vi "rsidr_core_global.vi"() -> ()   [LabVIEW 2015, in "Rohde&Schwarz CMXP Base.lvlib"]
doc: "This Global variable contains driver's:\n- Attributes\n- Range Tables\n- Repeated Capabilities"
uses:
  <instrlib>/Rohde&Schwarz CMXP Base/Rohde&Schwarz CMXP Base.lvlib
  <instrlib>/Rohde&Schwarz CMXP Base/Private/rsidr_core.llb/type_Input_Format_Attribute.ctl
  <instrlib>/Rohde&Schwarz CMXP Base/Private/rsidr_core.llb/type_Input_Format_RangeTable.ctl
  <instrlib>/Rohde&Schwarz CMXP Base/Private/rsidr_core.llb/type_Input_Format_RepCap.ctl
  <instrlib>/Rohde&Schwarz CMXP Base/Private/rsidr_core.llb/rsidr_core.lvlib
panel:
  in  "Repeated Capabilities":T1[](array[typedef])=[{"repCapName"="i", "indetifiers"=["chan1", "chan2", "chan3", "chan4", "chan5", "chan6", "chan7", "chan8", "chan9", "chan10", "chan11", "chan12", "chan13", "chan14", "chan15", "chan16", "chan17", "chan18", "chan19", "chan20", "chan21", "chan22", "chan23", "chan24", "chan25", "chan26", "chan27", "chan28", "chan29", "chan30", "chan31", "chan32"], "cmdValues"=["1", "2", "3", "4", "5", "6", "7", "8", "9", "10", "11", "12", "13", "14", "15", "16", "17", "18", "19", "20", "21", "22", "23", "24", "25", "26", "27", "28", "29", "30", "31", "32"]}]
  in  "Range Tables":T2[](array[typedef])=[{"Type"=2, "Name"="rsCmxpBase_rngMeasurementMode", "Entries"=[{"Name"="IQ", "Value 1"=0.0, "Value 2"=0.0, "Command"="IQ"}, {"Name"="Level", "Value 1"=1.0, "Value 2"=0.0, "Command"="LEV"}, {"Name"="Verify IQ", "Value 1"=2.0, "Value 2"=0.0, "Command"="VIQ"}]}, {"Type"=2, "Name"="rsCmxpBase_rngMode", "Entries"=[{"Name"="All", "Value 1"=0.0, "Value 2"=0.0, "Command"="ALL"}, {"Name"="Wtime", "Value 1"=1.0, "Value 2"=0.0, "Command"="WTI"}]}, {"Type"=2, "Name"="rsCmxpBase_rngOptionType", "Entries"=[{"Name"="All", "Value 1"=0.0, "Value 2"=0.0, "Command"="ALL"}, {"Name"="SW Option", "Value 1"=1.0, "Value 2"=0.0, "Command"="SWOP"}, {"Name"="HW Option", "Value 1"=2.0, "Value 2"=0.0, "Command"="HWOP"}, {"Name"="SW Package", "Value 1"=3.0, "Value 2"=0.0, "Command"="SWP"}, {"Name"="FWA", "Value 1"=4.0, "Value 2"=0.0, "Command"="FWA"}]}, {"Type"=2, "Name"="rsCmxpBase_rngValidity", "Entries"=[{"Name"="All", "Value 1"=0.0, "Value 2"=0.0, "Command"="ALL"}, {"Name"="Valid", "Value 1"=1.0, "Value 2"=0.0, "Command"="VAL"}, {"Name"="Functional", "Value 1"=2.0, "Value 2"=0.0, "Command"="FUNC"}]}, {"Type"=0, "Name"="rsCmxpBase_rngPortNumber", "Entries"=[{"Name"="", "Value 1"=0.0, "Value 2"=32767.0, "Command"=""}]}, {"Type"=0, "Name"="rsCmxpBase_rngTimer", "Entries"=[{"Name"="", "Value 1"=0.0, "Value 2"=inf, "Command"=""}]}, {"Type"=2, "Name"="rsCmxpBase_rngAuthenticationAlgorithm", "Entries"=[{"Name"="Milenage", "Value 1"=0.0, "Value 2"=0.0, "Command"="MIL"}, {"Name"="XOR", "Value 1"=1.0, "Value 2"=0.0, "Command"="XOR"}]}, {"Type"=2, "Name"="rsCmxpBase_rngOperatorCode", "Entries"=[{"Name"="Ciphered", "Value 1"=0.0, "Value 2"=0.0, "Command"="CIPH"}, {"Name"="Plain", "Value 1"=1.0, "Value 2"=0.0, "Command"="PLA"}]}, {"Type"=2, "Name"="rsCmxpBase_rngSelectFrequencyFormat", "Entries"=[{"Name"="Internal", "Value 1"=0.0, "Value 2"=0.0, "Command"="INTernal"}, {"Name"="External", "Value 1"=1.0, "Value 2"=0.0, "Command"="EXTernal"}]}, {"Type"=0, "Name"="rsCmxpBase_rngReferenceFrequencySettings", "Entries"=[{"Name"="", "Value 1"=1000000.0, "Value 2"=80000000.0, "Command"=""}]}, {"Type"=2, "Name"="rsCmxpBase_rngProtocolMode", "Entries"=[{"Name"="Raw", "Value 1"=0.0, "Value 2"=0.0, "Command"="RAW"}, {"Name"="Agilent", "Value 1"=1.0, "Value 2"=0.0, "Command"="AGIL"}, {"Name"="IEEE1147", "Value 1"=2.0, "Value 2"=0.0, "Command"="IEEE1174"}]}, {"Type"=2, "Name"="rsCmxpBase_rngQueryMeasurementState", "Entries"=[{"Name"="Off", "Value 1"=0.0, "Value 2"=0.0, "Command"="OFF"}, {"Name"="Run", "Value 1"=1.0, "Value 2"=0.0, "Command"="RUN"}, {"Name"="Ready", "Value 1"=2.0, "Value 2"=0.0, "Command"="RDY"}]}, {"Type"=2, "Name"="rsCmxpBase_rngQueryLastMeasurmentMode", "Entries"=[{"Name"="Invalid", "Value 1"=0.0, "Value 2"=0.0, "Command"="INV"}, {"Name"="Passed", "Value 1"=1.0, "Value 2"=0.0, "Command"="PASS"}, {"Name"="Progress", "Value 1"=2.0, "Value 2"=0.0, "Command"="PROG"}, {"Name"="Failed", "Value 1"=3.0, "Value 2"=0.0, "Command"="FAIL"}, {"Name"="Skipped", "Value 1"=4.0, "Value 2"=0.0, "Command"="SKIP"}, {"Name"="Not A Value", "Value 1"=5.0, "Value 2"=0.0, "Command"="NAV"}]}, {"Type"=2, "Name"="rsCmxpBase_rngRemoteTraceHeaderFilter", "Entries"=[{"Name"="All", "Value 1"=0.0, "Value 2"=0.0, "Command"="ALL"}, {"Name"="Line ID", "Value 1"=1.0, "Value 2"=0.0, "Command"="LID"}, {"Name"="Event Yype", "Value 1"=2.0, "Value 2"=0.0, "Command"="ETYP"}, {"Name"="Time Stamp", "Value 1"=3.0, "Value 2"=0.0, "Command"="TST"}, {"Name"="Duration", "Value 1"=4.0, "Value 2"=0.0, "Command"="DUR"}, {"Name"="VISA Resource", "Value 1"=5.0, "Value 2"=0.0, "Command"="VRES"}, {"Name"="Instrument Number", "Value 1"=6.0, "Value 2"=0.0, "Command"="TENV"}, {"Name"="Connection", "Value 1"=7.0, "Value 2"=0.0, "Command"="CONN"}, {"Name"="Data", "Value 1"=8.0, "Value 2"=0.0, "Command"="DATA"}]}, {"Type"=2, "Name"="rsCmxpBase_rngRemoteTraceTarget", "Entries"=[{"Name"="Screen", "Value 1"=0.0, "Value 2"=0.0, "Command"="SCR"}, {"Name"="File", "Value 1"=1.0, "Value 2"=0.0, "Command"="FILE"}, {"Name"="Screen and file", "Value 1"=2.0, "Value 2"=0.0, "Command"="SAF"}]}, {"Type"=2, "Name"="rsCmxpBase_rngDUTBandRestrictionTXConnector", "Entries"=[{"Name"="None", "Value 1"=0.0, "Value 2"=0.0, "Command"="NONE"}, {"Name"="One", "Value 1"=1.0, "Value 2"=0.0, "Command"="ONE"}]}, {"Type"=2, "Name"="rsCmxpBase_rngDUTBandRestrictionRXConnector", "Entries"=[{"Name"="None", "Value 1"=0.0, "Value 2"=0.0, "Command"="NONE"}, {"Name"="One", "Value 1"=1.0, "Value 2"=0.0, "Command"="ONE"}, {"Name"="Two", "Value 1"=2.0, "Value 2"=0.0, "Command"="TWO"}]}, {"Type"=2, "Name"="rsCmxpBase_rngDUTControlMode", "Entries"=[{"Name"="Manual", "Value 1"=0.0, "Value 2"=0.0, "Command"="MAN"}, {"Name"="Automatic", "Value 1"=1.0, "Value 2"=0.0, "Command"="AUTO"}]}, {"Type"=2, "Name"="rsCmxpBase_rngUSIMLengthXOR", "Entries"=[{"Name"="Any", "Value 1"=0.0, "Value 2"=0.0, "Command"="ANY"}, {"Name"="L04", "Value 1"=1.0, "Value 2"=0.0, "Command"="L04"}, {"Name"="L05", "Value 1"=2.0, "Value 2"=0.0, "Command"="L05"}, {"Name"="L06", "Value 1"=3.0, "Value 2"=0.0, "Command"="L06"}, {"Name"="L07", "Value 1"=4.0, "Value 2"=0.0, "Command"="L07"}, {"Name"="L08", "Value 1"=5.0, "Value 2"=0.0, "Command"="L08"}, {"Name"="L09", "Value 1"=6.0, "Value 2"=0.0, "Command"="L09"}, {"Name"="L10", "Value 1"=7.0, "Value 2"=0.0, "Command"="L10"}, {"Name"="L11", "Value 1"=8.0, "Value 2"=0.0, "Command"="L11"}, {"Name"="L12", "Value 1"=9.0, "Value 2"=0.0, "Command"="L12"}, {"Name"="L13", "Value 1"=10.0, "Value 2"=0.0, "Command"="L13"}, {"Name"="L14", "Value 1"=11.0, "Value 2"=0.0, "Command"="L14"}, {"Name"="L15", "Value 1"=12.0, "Value 2"=0.0, "Command"="L15"}, {"Name"="L16", "Value 1"=13.0, "Value 2"=0.0, "Command"="L16"}]}, {"Type"=2, "Name"="rsCmxpBase_rngDUTPowerCycleState", "Entries"=[{"Name"="Ready", "Value 1"=0.0, "Value 2"=0.0, "Command"="RDY"}, {"Name"="Run", "Value 1"=1.0, "Value 2"=0.0, "Command"="RUN"}]}, {"Type"=2, "Name"="rsCmxpBase_rngDataFormat", "Entries"=[{"Name"="ASCII", "Value 1"=0.0, "Value 2"=0.0, "Command"="ASC"}, {"Name"="Real", "Value 1"=1.0, "Value 2"=0.0, "Command"="REAL"}, {"Name"="Binary", "Value 1"=2.0, "Value 2"=0.0, "Command"="BIN"}, {"Name"="Hexadecimal", "Value 1"=3.0, "Value 2"=0.0, "Command"="HEX"}, {"Name"="Octal", "Value 1"=4.0, "Value 2"=0.0, "Command"="OCT"}]}, {"Type"=2, "Name"="rsCmxpBase_rngSeverity", "Entries"=[{"Name"="Info", "Value 1"=0.0, "Value 2"=0.0, "Command"="INFO"}, {"Name"="Warning", "Value 1"=1.0, "Value 2"=0.0, "Command"="WARN"}, {"Name"="Error", "Value 1"=2.0, "Value 2"=0.0, "Command"="ERR"}]}, {"Type"=2, "Name"="rsCmxpBase_rngTriggerDirection", "Entries"=[{"Name"="In", "Value 1"=0.0, "Value 2"=0.0, "Command"="IN"}, {"Name"="Out", "Value 1"=1.0, "Value 2"=0.0, "Command"="OUT"}]}, {"Type"=2, "Name"="rsCmxpBase_rngTriggerSlope", "Entries"=[{"Name"="Rising Edge", "Value 1"=0.0, "Value 2"=0.0, "Command"="REDG"}, {"Name"="Falling Edge", "Value 1"=1.0, "Value 2"=0.0, "Command"="FEDG"}]}, {"Type"=2, "Name"="rsCmxpBase_rngTriggerConnectorCatalogNameStyle", "Entries"=[{"Name"="Default", "Value 1"=0.0, "Value 2"=0.0, "Command"="NAME"}, {"Name"="Fully Qualified Name", "Value 1"=1.0, "Value 2"=0.0, "Command"="FQN"}, {"Name"="Label Only", "Value 1"=2.0, "Value 2"=0.0, "Command"="LNAM"}]}, {"Type"=2, "Name"="rsCmxpBase_rngDUTBandRestrictionType", "Entries"=[{"Name"="LTE", "Value 1"=0.0, "Value 2"=0.0, "Command"="LTE"}, {"Name"="New Radio", "Value 1"=1.0, "Value 2"=0.0, "Command"="NRAD"}]}, {"Type"=2, "Name"="rsCmxpBase_rngDUTBandTX", "Entries"=[{"Name"="TX0", "Value 1"=0.0, "Value 2"=0.0, "Command"="TX0"}, {"Name"="TX1", "Value 1"=1.0, "Value 2"=0.0, "Command"="TX1"}, {"Name"="None", "Value 1"=2.0, "Value 2"=0.0, "Command"="NONE"}]}, {"Type"=2, "Name"="rsCmxpBase_rngDUTBandRX", "Entries"=[{"Name"="RX0", "Value 1"=0.0, "Value 2"=0.0, "Command"="RX0"}, {"Name"="RX1", "Value 1"=1.0, "Value 2"=0.0, "Command"="RX1"}, {"Name"="RX2", "Value 1"=2.0, "Value 2"=0.0, "Command"="RX2"}, {"Name"="RX3", "Value 1"=3.0, "Value 2"=0.0, "Command"="RX3"}, {"Name"="None", "Value 1"=4.0, "Value 2"=0.0, "Command"="NONE"}]}, {"Type"=2, "Name"="rsCmxpBase_rngDUTBandType", "Entries"=[{"Name"="LTE", "Value 1"=0.0, "Value 2"=0.0, "Command"="LTE"}, {"Name"="New Radio", "Value 1"=1.0, "Value 2"=0.0, "Command"="NRAD"}, {"Name"="WLAN", "Value 1"=2.0, "Value 2"=0.0, "Command"="WLAN"}]}, {"Type"=2, "Name"="rsCmxpBase_rngDUTControlAutomationFramework", "Entries"=[{"Name"="External Automation Application", "Value 1"=0.0, "Value 2"=0.0, "Command"="EXT"}]}, {"Type"=2, "Name"="rsCmxpBase_rngRemoteTraceLogRows", "Entries"=[{"Name"="Latest", "Value 1"=0.0, "Value 2"=0.0, "Command"="LAT"}, {"Name"="List", "Value 1"=1.0, "Value 2"=0.0, "Command"="LIST"}, {"Name"="Error", "Value 1"=2.0, "Value 2"=0.0, "Command"="ERR"}, {"Name"="Connection", "Value 1"=3.0, "Value 2"=0.0, "Command"="CONN"}]}, {"Type"=2, "Name"="rsCmxpBase_rngRemoteTraceEvents", "Entries"=[{"Name"="All", "Value 1"=0.0, "Value 2"=0.0, "Command"="ALL"}, {"Name"="Input", "Value 1"=1.0, "Value 2"=0.0, "Command"="INP"}, {"Name"="Output", "Value 1"=2.0, "Value 2"=0.0, "Command"="OUTP"}, {"Name"="Error", "Value 1"=3.0, "Value 2"=0.0, "Command"="ERR"}, {"Name"="Connection", "Value 1"=4.0, "Value 2"=0.0, "Command"="CONN"}, {"Name"="Duration", "Value 1"=5.0, "Value 2"=0.0, "Command"="DUR"}, {"Name"="Remote Local", "Value 1"=6.0, "Value 2"=0.0, "Command"="RLOC"}]}, {"Type"=2, "Name"="rsCmxpBase_rngRFConnectionDirection", "Entries"=[{"Name"="RX", "Value 1"=0.0, "Value 2"=0.0, "Command"="RX"}, {"Name"="TX", "Value 1"=1.0, "Value 2"=0.0, "Command"="TX"}, {"Name"="TX & RX", "Value 1"=2.0, "Value 2"=0.0, "Command"="RXTX"}]}, {"Type"=0, "Name"="rsCmxpBase_rngSystemDataFormat", "Entries"=[{"Name"="", "Value 1"=0.0, "Value 2"=0.0, "Command"=""}]}, {"Type"=2, "Name"="rsCmxpBase_rngActiveDUTActionState", "Entries"=[{"Name"="Ready", "Value 1"=0.0, "Value 2"=0.0, "Command"="RDY"}, {"Name"="Run", "Value 1"=1.0, "Value 2"=0.0, "Command"="RUN"}]}, {"Type"=2, "Name"="rsCmxpBase_rngActiveDUTMobileAction", "Entries"=[{"Name"="Reject", "Value 1"=0.0, "Value 2"=0.0, "Command"="REJ"}, {"Name"="Disconnect", "Value 1"=1.0, "Value 2"=0.0, "Command"="DISC"}, {"Name"="Accept", "Value 1"=2.0, "Value 2"=0.0, "Command"="ACC"}, {"Name"="Connect", "Value 1"=3.0, "Value 2"=0.0, "Command"="CONN"}]}] {"Type" items=["Range", "Coerced", "Discrete"]}
  in  "Attributes":T3[](array[typedef])=[{"Level"=1, "Class Only"=TRUE, "Identifier"="", "Descriptive Name"="Base", "Data Type"=0, "Command"="", "Access"=0, "Range Table"="", "Read Callback"="", "Write Callback"="", "Supported Models"="", "Instrument Options"="", "Flags"=0, "Help"="Contains functionality to configure the base R&S Radio Communication Tester."}, {"Level"=2, "Class Only"=TRUE, "Identifier"="", "Descriptive Name"="Macro", "Data Type"=0, "Command"="", "Access"=0, "Range Table"="", "Read Callback"="", "Write Callback"="", "Supported Models"="", "Instrument Options"="", "Flags"=0, "Help"="The following remote control commands are related to macro files and macro execution."}, {"Level"=3, "Class Only"=FALSE, "Identifier"="RSCMXPBASE_ATTR_CREATE_MACRO", "Descriptive Name"="Create Macro", "Data Type"=6, "Command"="*DMC", "Access"=2, "Range Table"="", "Read Callback"="", "Write Callback"="", "Supported Models"="", "Instrument Options"="", "Flags"=0, "Help"="Creates a macro. If the label exists already, the macro contents are overwritten. Macros are deleted when a remote connection is closed but can be saved to a macro file for later reuse, see MMEMory:STORe:MACRo. Avoid using labels which are identical with supported remote control commands.  In contrast to SCPI stipulations, remote commands have priority over macros.\n\nAvailable Repeated Capabilities:\nNone\n\nRemote-control command(s):\n*DMC"}, {"Level"=3, "Class Only"=FALSE, "Identifier"="RSCMXPBASE_ATTR_MACRO_EXECUTION_STATE", "Descriptive Name"="Macro Execution State", "Data Type"=3, "Command"="*EMC", "Access"=2, "Range Table"="", "Read Callback"="", "Write Callback"="", "Supported Models"="", "Instrument Options"="", "Flags"=0, "Help"="Enables or disables the execution of all macros that are defined for the active remote connection. Note: In contrast to SCPI specifications, macro execution is disabled by default.\n\nAvailable Repeated Capabilities:\nNone\n\nRemote-control command(s):\n*EMC"}, {"Level"=3, "Class Only"=FALSE, "Identifier"="RSCMXPBASE_ATTR_HIDDEN_QUERY_MACRO", "Descriptive Name"="Query Macro", "Data Type"=2, "Command"="*GMC?", "Access"=0, "Range Table"="", "Read Callback"="", "Write Callback"="", "Supported Models"="", "Instrument Options"="", "Flags"=8, "Help"="Returns the contents of a macro.\n\nAvailable Repeated Capabilities:\nNone\n\nRemote-control command(s):\n*GMC?"}, {"Level"=3, "Class Only"=FALSE, "Identifier"="RSCMXPBASE_ATTR_QUERY_MACRO_LABELS", "Descriptive Name"="Query Macro Labels", "Data Type"=2, "Command"="*LMC?", "Access"=0, "Range Table"="", "Read Callback"="", "Write Callback"="", "Supported Models"="", "Instrument Options"="", "Flags"=0, "Help"="Returns the labels of all macros of the active connection.\n\nAvailable Repeated Capabilities:\nNone\n\nRemote-control command(s):\n*LMC?"}, {"Level"=3, "Class Only"=FALSE, "Identifier"="RSCMXPBASE_ATTR_DELETE_ALL_MACROS", "Descriptive Name"="Delete All Macros", "Data Type"=4, "Command"="*PMC", "Access"=1, "Range Table"="", "Read Callback"="", "Write Callback"="", "Supported Models"="", "Instrument Options"="", "Flags"=0, "Help"="Deletes all macros of the active remote connection.\n\nAvailable Repeated Capabilities:\nNone\n\nRemote-control command(s):\n*PMC"}, {"Level"=3, "Class Only"=FALSE, "Identifier"="RSCMXPBASE_ATTR_DELETE_MACRO", "Descriptive Name"="Delete Macro", "Data Type"=2, "Command"="*RMC", "Access"=1, "Range Table"="", "Read Callback"="", "Write Callback"="", "Supported Models"="", "Instrument Options"="", "Flags"=0, "Help"="Deletes a macro.\n\nAvailable Repeated Capabilities:\nNone\n\nRemote-control command(s):\n*RMC"}, {"Level"=3, "Class Only"=FALSE, "Identifier"="RSCMXPBASE_ATTR_LOAD_MACRO", "Descriptive Name"="Load Macro", "Data Type"=6, "Command"="MMEM:LOAD:MACR", "Access"=2, "Range Table"="", "Read Callback"="", "Write Callback"="", "Supported Models"="", "Instrument Options"="", "Flags"=0, "Help"="Creates a macro, reading the macro contents from a file. If the label exists already, the macro contents are overwritten.\nAvoid using labels which are identical with supported remote control commands.  In contrast to SCPI stipulations, remote commands have priority over macros.\n\nAvailable Repeated Capabilities:\nNone\n\nRemote-control command(s):\nMMEMory:LOAD:MACRo"}, {"Level"=3, "Class Only"=FALSE, "Identifier"="RSCMXPBASE_ATTR_SAVE_MACRO", "Descriptive Name"="Save Macro", "Data Type"=6, "Command"="MMEM:STOR:MACR", "Access"=1, "Range Table"="", "Read Callback"="", "Write Callback"="", "Supported Models"="", "Instrument Options"="", "Flags"=0, "Help"="Stores the contents of a macro to a file. If the file exists, it is overwritten. If the file does not exist, it is created.\n\nAvailable Repeated Capabilities:\nNone\n\nRemote-control command(s):\nMMEMory:STORe:MACRo"}, {"Level"=3, "Class Only"=FALSE, "Identifier"="RSCMXPBASE_ATTR_START_MACRO_RECORDING", "Descriptive Name"="Start Macro Recording", "Data Type"=2, "Command"="SYST:REC:MACR:FILE:STAR", "Access"=1, "Range Table"="", "Read Callback"="", "Write Callback"="", "Supported Models"="", "Instrument Options"="", "Flags"=0, "Help"="Starts recording of submitted commands into a macro file. If the file exists, it is overwritten. If the file does not exist, it is created.\n\nAvailable Repeated Capabilities:\nNone\n\nRemote-control command(s):\nSYSTem:RECord:MACRo:FILE:STARt"}, {"Level"=3, "Class Only"=FALSE, "Identifier"="RSCMXPBASE_ATTR_STOP_MACRO_RECORDING", "Descriptive Name"="Stop Macro Recording", "Data Type"=4, "Command"="SYST:REC:MACR:FILE:STOP", "Access"=1, "Range Table"="", "Read Callback"="", "Write Callback"="", "Supported Models"="", "Instrument Options"="", "Flags"=0, "Help"="Stops recording of commands into a macro file.\n\nAvailable Repeated Capabilities:\nNone\n\nRemote-control command(s):\nSYSTem:RECord:MACRo:FILE:STOP"}, {"Level"=2, "Class Only"=TRUE, "Identifier"="", "Descriptive Name"="Buffer", "Data Type"=0, "Command"="", "Access"=0, "Range Table"="", "Read Callback"="", "Write Callback"="", "Supported Models"="", "Instrument Options"="", "Flags"=0, "Help"="The following remote control commands are related to response buffers."}, {"Level"=3, "Class Only"=FALSE, "Identifier"="RSCMXPBASE_ATTR_START_BUFFER", "Descriptive Name"="Start Buffer", "Data Type"=2, "Command"="STAR:BASE:BUFF", "Access"=1, "Range Table"="", "Read Callback"="", "Write Callback"="", "Supported Models"="", "Instrument Options"="", "Flags"=0, "Help"="Creates and activates a buffer. If the buffer exists already, it is cleared (equivalent to CLEar:BASE:BUFFer).\n\nAvailable Repeated Capabilities:\nNone\n\nRemote-control command(s):\nSTARt:BASE:BUFFer"}, {"Level"=3, "Class Only"=FALSE, "Identifier"="RSCMXPBASE_ATTR_STOP_BUFFER", "Descriptive Name"="Stop Buffer", "Data Type"=4, "Command"="STOP:BASE:BUFF", "Access"=1, "Range Table"="", "Read Callback"="", "Write Callback"="", "Supported Models"="", "Instrument Options"="", "Flags"=0, "Help"="Deactivates the active buffer. Only one buffer can be active at a time. The buffer and its contents are maintained, but data recording is paused. Use CONTinue:BASE:BUFFer to reactivate a buffer.\n\nAvailable Repeated Capabilities:\nNone\n\nRemote-control command(s):\nSTOP:BASE:BUFFer"}, {"Level"=3, "Class Only"=FALSE, "Identifier"="RSCMXPBASE_ATTR_CONTINUE_BUFFER", "Descriptive Name"="Continue Buffer", "Data Type"=2, "Command"="CONT:BASE:BUFF", "Access"=1, "Range Table"="", "Read Callback"="", "Write Callback"="", "Supported Models"="", "Instrument Options"="", "Flags"=0, "Help"="Reactivates a buffer which was deactivated via STOP:BASE:BUFFer). The R&S CMX500 continues writing data to the buffer.\n\nAvailable Repeated Capabilities:\nNone\n\nRemote-control command(s):\nCONTinue:BASE:BUFFer"}, {"Level"=3, "Class Only"=FALSE, "Identifier"="RSCMXPBASE_ATTR_HIDDEN_FETCH_BUFFER", "Descriptive Name"="Fetch Buffer", "Data Type"=6, "Command"="FETC:BASE:BUFF?", "Access"=0, "Range Table"="", "Read Callback"="", "Write Callback"="", "Supported Models"="", "Instrument Options"="", "Flags"=8, "Help"="Reads the contents of a buffer line. Buffer contents are stored line by line. Every query generates a new buffer line. The queries are not stored together with the results. Reading buffer contents is non-destructive. The lines can be read in arbitrary order.\n\nAvailable Repeated Capabilities:\nNone\n\nRemote-control command(s):\nFETCh:BASE:BUFFer?"}, {"Level"=3, "Class Only"=FALSE, "Identifier"="RSCMXPBASE_ATTR_HIDDEN_FETCH_BUFFER_LINES", "Descriptive Name"="Fetch Buffer Lines", "Data Type"=0, "Command"="FETC:BASE:BUFF:LIN?", "Access"=0, "Range Table"="", "Read Callback"="", "Write Callback"="", "Supported Models"="", "Instrument Options"="", "Flags"=8, "Help"="Returns the number of lines in a buffer.\n\nAvailable Repeated Capabilities:\nNone\n\nRemote-control command(s):\nFETCh:BASE:BUFFer:LINecount?"}, {"Level"=3, "Class Only"=FALSE, "Identifier"="RSCMXPBASE_ATTR_CLEAR_BUFFER", "Descriptive Name"="Clear Buffer", "Data Type"=2, "Command"="CLE:BASE:BUFF", "Access"=1, "Range Table"="", "Read Callback"="", "Write Callback"="", "Supported Models"="", "Instrument Options"="", "Flags"=0, "Help"="Clears the contents of a buffer. You get an empty buffer that you can fill with new commands.\n\nAvailable Repeated Capabilities:\nNone\n\nRemote-control command(s):\nCLEar:BASE:BUFFer"}, {"Level"=3, "Class Only"=FALSE, "Identifier"="RSCMXPBASE_ATTR_DELETE_BUFFER", "Descriptive Name"="Delete Buffer", "Data Type"=2, "Command"="DEL:BASE:BUFF", "Access"=1, "Range Table"="", "Read Callback"="", "Write Callback"="", "Supported Models"="", "Instrument Options"="", "Flags"=0, "Help"="Deletes a buffer.\n\nAvailable Repeated Capabilities:\nNone\n\nRemote-control command(s):\nDELete:BASE:BUFFer"}, {"Level"=2, "Class Only"=TRUE, "Identifier"="", "Descriptive Name"="Timer", "Data Type"=0, "Command"="", "Access"=0, "Range Table"="", "Read Callback"="", "Write Callback"="", "Supported Models"="", "Instrument Options"="", "Flags"=0, "Help"="After execution of a command, it can be necessary to wait a well-defined time before proceeding with command script processing. For example, because the DUT needs some time to stabilize after a modification. Waiting can be achieved using the following commands."}, {"Level"=3, "Class Only"=FALSE, "Identifier"="RSCMXPBASE_ATTR_SET_ABSOLUTE_TIMER", "Descriptive Name"="Set Absolute Timer", "Data Type"=0, "Command"="SYST:TIME:HRT:ABS", "Access"=1, "Range Table"="rsCmxpBase_rngTimer", "Read Callback"="", "Write Callback"="", "Supported Models"="", "Instrument Options"="", "Flags"=1, "Help"="Starts a timer. The timeout is specified relative to an already set timestamp, see RSCMXPBASE_ATTR_SET_TIMESTAMP. When the timer expires, 'Operation Complete' is indicated. This event can be evaluated by polling, via a *OPC? or via *WAI.\n\nAvailable Repeated Capabilities:\nNone\n\nRemote-control command(s):\nSYSTem:TIME:HRTimer:ABSolute"}, {"Level"=3, "Class Only"=FALSE, "Identifier"="RSCMXPBASE_ATTR_SET_RELATIVE_TIMER", "Descriptive Name"="Set Relative Timer", "Data Type"=0, "Command"="SYST:TIME:HRT:REL", "Access"=1, "Range Table"="rsCmxpBase_rngTimer", "Read Callback"="", "Write Callback"="", "Supported Models"="", "Instrument Options"="", "Flags"=1, "Help"="Starts a timer. After the specified timeout, an OPC is generated. When the timer expires, 'Operation Complete' is indicated. This event can be evaluated by polling, via a *OPC? or via *WAI.\n\nAvailable Repeated Capabilities:\nNone\n\nRemote-control command(s):\nSYSTem:TIME:HRTimer:RELative"}, {"Level"=3, "Class Only"=FALSE, "Identifier"="RSCMXPBASE_ATTR_SET_TIMESTAMP", "Descriptive Name"="Set Timestamp", "Data Type"=4, "Command"="SYST:TIME:HRT:ABS:SET", "Access"=1, "Range Table"="", "Read Callback"="", "Write Callback"="", "Supported Models"="", "Instrument Options"="", "Flags"=0, "Help"="This command sets a timestamp with the current system time. A timer can be started with a timeout relative to this timestamp, see SYSTem:TIME:HRTimer:ABSolute. An existing timestamp is overwritten.\n\nAvailable Repeated Capabilities:\nNone\n\nRemote-control command(s):\nSYSTem:TIME:HRTimer:ABSolute:SET"}, {"Level"=3, "Class Only"=FALSE, "Identifier"="RSCMXPBASE_ATTR_QUERY_TIMESTAMP", "Descriptive Name"="Query Timestamp", "Data Type"=2, "Command"="SYST:TIME:HRT:ABS:SET?", "Access"=0, "Range Table"="", "Read Callback"="", "Write Callback"="", "Supported Models"="", "Instrument Options"="", "Flags"=0, "Help"="This command queries a timestamp with the current system time. A query returns seven values, separated by commas:\nYear, month, day, hour, minutes, seconds, milliseconds\n\nAvailable Repeated Capabilities:\nNone\n\nRemote-control command(s):\nSYSTem:TIME:HRTimer:ABSolute:SET?"}, {"Level"=2, "Class Only"=TRUE, "Identifier"="", "Descriptive Name"="DUT", "Data Type"=0, "Command"="", "Access"=0, "Range Table"="", "Read Callback"="", "Write Callback"="", "Supported Models"="", "Instrument Options"="", "Flags"=0, "Help"="Contains settings related to DUTs. Additional DUT settings directly related to signaling are described in the signaling manual.\n\nPrepare DUTs in the library and use exactly one active DUT in the test environment."}, {"Level"=3, "Class Only"=TRUE, "Identifier"="", "Descriptive Name"="Library", "Data Type"=0, "Command"="", "Access"=0, "Range Table"="", "Read Callback"="", "Write Callback"="", "Supported Models"="", "Instrument Options"="", "Flags"=0, "Help"="Contains settings for managing DUTs in a library.\n\nA DUT object has a name, SIM slots, a referenced SIM profile per SIM slot and antenna connectors supporting certain frequency bands."}, {"Level"=4, "Class Only"=FALSE, "Identifier"="RSCMXPBASE_ATTR_DUT_CATALOG", "Descriptive Name"="DUT Catalog", "Data Type"=2, "Command"="CAT:DUT?", "Access"=0, "Range Table"="", "Read Callback"="", "Write Callback"="", "Supported Models"="", "Instrument Options"="", "Flags"=0, "Help"="Queries a list of all DUTs, including inactive DUTs in the library and the active DUT.\n\nAvailable Repeated Capabilities:\nNone\n\nRemote-control command(s):\nCATalog:DUT?"}, {"Level"=4, "Class Only"=FALSE, "Identifier"="RSCMXPBASE_ATTR_DUT_ADD", "Descriptive Name"="DUT Add", "Data Type"=2, "Command"="CRE:DUT", "Access"=1, "Range Table"="", "Read Callback"="", "Write Callback"="", "Supported Models"="", "Instrument Options"="", "Flags"=0, "Help"="Creates a DUT with the specified name.\n\nAssign a unique name to each named object within the test environment. Assigning an already used name can be rejected with an error message, even if the other object has not the same type as the new object.\n\nAvailable Repeated Capabilities:\nNone\n\nRemote-control command(s):\nCREate:DUT"}, {"Level"=4, "Class Only"=FALSE, "Identifier"="RSCMXPBASE_ATTR_HIDDEN_DUT_DUPLICATE", "Descriptive Name"="Hidden DUT Duplicate", "Data Type"=6, "Command"="COPY:DUT", "Access"=1, "Range Table"="", "Read Callback"="", "Write Callback"="", "Supported Models"="", "Instrument Options"="", "Flags"=8, "Help"="Creates a DUT with a new name as a copy of the DUT specified.\n\nAvailable Repeated Capabilities:\nNone\n\nRemote-control command(s):\nCOPY:DUT"}, {"Level"=4, "Class Only"=FALSE, "Identifier"="RSCMXPBASE_ATTR_DUT_DELETE", "Descriptive Name"="DUT Delete", "Data Type"=2, "Command"="DEL:DUT", "Access"=1, "Range Table"="", "Read Callback"="", "Write Callback"="", "Supported Models"="", "Instrument Options"="", "Flags"=0, "Help"="Deletes the DUT with the specified name.\n\nAvailable Repeated Capabilities:\nNone\n\nRemote-control command(s):\nDELete:DUT"}, {"Level"=4, "Class Only"=TRUE, "Identifier"="", "Descriptive Name"="Bands And Connectors", "Data Type"=0, "Command"="", "Access"=0, "Range Table"="", "Read Callback"="", "Write Callback"="", "Supported Models"="", "Instrument Options"="", "Flags"=0, "Help"="Configures the antenna connectors of the inactive DUTs."}, {"Level"=5, "Class Only"=FALSE, "Identifier"="RSCMXPBASE_ATTR_HIDDEN_DUT_CONNECTOR_ADD", "Descriptive Name"="Hidden DUT Connector Add", "Data Type"=6, "Command"="CRE:DUT:PROF:CONN", "Access"=1, "Range Table"="", "Read Callback"="", "Write Callback"="", "Supported Models"="", "Instrument Options"="", "Flags"=8, "Help"="Creates an antenna connector for the inactive DUT.\n\nAssign a unique name to each named object within the test environment. Assigning an already used name can be rejected with an error message, even if the other object has not the same type as the new object.\n\nAvailable Repeated Capabilities:\nNone\n\nRemote-control command(s):\nCREate:DUT:PROFile:CONNector"}, {"Level"=5, "Class Only"=FALSE, "Identifier"="RSCMXPBASE_ATTR_HIDDEN_DUT_CONNECTOR_DELETE", "Descriptive Name"="Hidden DUT Connector Delete", "Data Type"=6, "Command"="DEL:DUT:PROF:CONN", "Access"=1, "Range Table"="", "Read Callback"="", "Write Callback"="", "Supported Models"="", "Instrument Options"="", "Flags"=8, "Help"="Deletes an antenna connector of the inactive DUT.\n\nAvailable Repeated Capabilities:\nNone\n\nRemote-control command(s):\nDELete:DUT:PROFile:CONNector"}, {"Level"=5, "Class Only"=FALSE, "Identifier"="RSCMXPBASE_ATTR_HIDDEN_DUT_CONNECTOR_CATALOG", "Descriptive Name"="Hidden DUT Connector Catalog", "Data Type"=6, "Command"="CAT:DUT:PROF:CONN?", "Access"=0, "Range Table"="", "Read Callback"="", "Write Callback"="", "Supported Models"="", "Instrument Options"="", "Flags"=8, "Help"="Queries a list of all antenna connectors of the inactive DUT.\n\nAvailable Repeated Capabilities:\nNone\n\nRemote-control command(s):\nCATalog:DUT:PROFile:CONNector?"}, {"Level"=5, "Class Only"=FALSE, "Identifier"="RSCMXPBASE_ATTR_HIDDEN_DUT_CONNECTOR_BAND_ADD", "Descriptive Name"="Hidden DUT Connector Band Add", "Data Type"=6, "Command"="ADD:DUT:PROF:CONN:BAND", "Access"=1, "Range Table"="", "Read Callback"="", "Write Callback"="", "Supported Models"="", "Instrument Options"="", "Flags"=8, "Help"="Assigns frequency bands to a single antenna connector of the inactive DUT (connector-centric approach).\n\nYou can assign several bands with a single command. Specify the technology and the band number for each band.\n\nAvailable Repeated Capabilities:\nNone\n\nRemote-control command(s):\nADD:DUT:PROFile:CONNector:BAND"}, {"Level"=5, "Class Only"=FALSE, "Identifier"="RSCMXPBASE_ATTR_HIDDEN_DUT_CONNECTOR_BAND_DELETE", "Descriptive Name"="Hidden DUT Connector Band Delete", "Data Type"=6, "Command"="REM:DUT:PROF:CONN:BAND", "Access"=1, "Range Table"="", "Read Callback"="", "Write Callback"="", "Supported Models"="", "Instrument Options"="", "Flags"=8, "Help"="Removes frequency bands from an antenna connector of the inactive DUT (connector-centric approach).\n\nYou can remove several bands. Specify the technology and the band number for each band.\n\nAvailable Repeated Capabilities:\nNone\n\nRemote-control command(s):\nREMove:DUT:PROFile:CONNector:BAND"}, {"Level"=5, "Class Only"=FALSE, "Identifier"="RSCMXPBASE_ATTR_HIDDEN_DUT_CONNECTOR_BAND_CATALOG", "Descriptive Name"="Hidden DUT Connector Band Catalog", "Data Type"=6, "Command"="CAT:DUT:PROF:CONN:BAND?", "Access"=0, "Range Table"="", "Read Callback"="", "Write Callback"="", "Supported Models"="", "Instrument Options"="", "Flags"=8, "Help"="Queries a list of all frequency bands assigned to an antenna connector of the inactive DUT. Structured according to the connector-centric approach.\n\nThe results are returned as groups of values, with <NoOfBands> pairs of <RatType>, <BandNumber> per group:\n\n{<TX>, <RX>, <NoOfBands>, {<RatType>, <BandNumber>,}<NoOfBands> times} ...\n\nAvailable Repeated Capabilities:\nNone\n\nRemote-control command(s):\nCATalog:DUT:PROFile:CONNector:BAND?"}, {"Level"=4, "Class Only"=TRUE, "Identifier"="", "Descriptive Name"="SIM Slot", "Data Type"=0, "Command"="", "Access"=0, "Range Table"="", "Read Callback"="", "Write Callback"="", "Supported Models"="", "Instrument Options"="", "Flags"=0, "Help"="Manage the SIM slots of inactive DUT objects."}, {"Level"=5, "Class Only"=FALSE, "Identifier"="RSCMXPBASE_ATTR_HIDDEN_DUT_SIM_SLOT_ADD", "Descriptive Name"="Hidden DUT SIM Slot Add", "Data Type"=6, "Command"="CRE:DUT:PROF:SIMS", "Access"=1, "Range Table"="", "Read Callback"="", "Write Callback"="", "Supported Models"="", "Instrument Options"="", "Flags"=8, "Help"="Adds a SIM slot with the assigned SIM profile name to the inactive DUT with the specified name.\n\nAssign a unique name to each named object within the test environment. Assigning an already used name can be rejected with an error message, even if the other object has not the same type as the new object.\n\nAvailable Repeated Capabilities:\nNone\n\nRemote-control command(s):\nCREate:DUT:PROFile:SIMSlot"}, {"Level"=5, "Class Only"=FALSE, "Identifier"="RSCMXPBASE_ATTR_HIDDEN_DUT_SIM_SLOT_DELETE", "Descriptive Name"="Hidden DUT SIM Slot Delete", "Data Type"=6, "Command"="DEL:DUT:PROF:SIMS", "Access"=1, "Range Table"="", "Read Callback"="", "Write Callback"="", "Supported Models"="", "Instrument Options"="", "Flags"=8, "Help"="Deletes the SIM slot with the specified SIM number from the inactive DUT.\n\nAvailable Repeated Capabilities:\nNone\n\nRemote-control command(s):\nDELete:DUT:PROFile:SIMSlot"}, {"Level"=5, "Class Only"=FALSE, "Identifier"="RSCMXPBASE_ATTR_HIDDEN_DUT_SIM_SLOT_CATALOG", "Descriptive Name"="Hidden DUT SIM Slot Catalog", "Data Type"=6, "Command"="CAT:DUT:PROF:SIMS?", "Access"=0, "Range Table"="", "Read Callback"="", "Write Callback"="", "Supported Models"="", "Instrument Options"="", "Flags"=8, "Help"="Queries all SIM slots of the inactive DUT. For each SIM slot, the number and the slot name are returned:\n\n{<SimSlotNo>, <SimProfileName>}1, {...}2, ...\n\nAvailable Repeated Capabilities:\nNone\n\nRemote-control command(s):\nCATalog:DUT:PROFile:SIMSlot?"}, {"Level"=5, "Class Only"=FALSE, "Identifier"="RSCMXPBASE_ATTR_SELECT_DUT_SIM_SLOT", "Descriptive Name"="Select DUT SIM Slot", "Data Type"=0, "Command"="", "Access"=2, "Range Table"="", "Read Callback"="", "Write Callback"="", "Supported Models"="", "Instrument Options"="", "Flags"=0, "Help"="Selects a SIM slot number.\n\nAvailable Repeated Capabilities:\nNone\n\nRemote-control command(s):\n"}, {"Level"=5, "Class Only"=FALSE, "Identifier"="RSCMXPBASE_ATTR_HIDDEN_DUT_SIM_SLOT_PROFILE", "Descriptive Name"="Hidden DUT SIM Slot Profile", "Data Type"=6, "Command"="DUT:PROF:SIMS<SIMSlot>:SIMP", "Access"=2, "Range Table"="", "Read Callback"="rscmxpbase_FormatSIMSlotRepCapRawString_ReadCallback.vi", "Write Callback"="rscmxpbase_FormatSIMSlotRepCapRawString_WriteCallback.vi", "Supported Models"="", "Instrument Options"="", "Flags"=8, "Help"="Assigns the SIM profile to the SlM slot number of the inactive DUT.\n\nAvailable Repeated Capabilities:\nNone\n\nRemote-control command(s):\n[CONFigure:]DUT:PROFile:SIMSlot<no>:SIMProfile"}, {"Level"=5, "Class Only"=FALSE, "Identifier"="RSCMXPBASE_ATTR_HIDDEN_DUT_SIM_SLOT_IMS_SUPPORTED", "Descriptive Name"="Hidden DUT SIM Slot IMS Supported", "Data Type"=6, "Command"="DUT:PROF:SIMS<SIMSlot>:CAP:IMS", "Access"=2, "Range Table"="", "Read Callback"="rscmxpbase_FormatSIMSlotRepCapRawString_ReadCallback.vi", "Write Callback"="rscmxpbase_FormatSIMSlotRepCapRawString_WriteCallback.vi", "Supported Models"="", "Instrument Options"="", "Flags"=8, "Help"="Selects whether the inactive DUT supports IP multimedia subsystem (IMS) services.\n\nAvailable Repeated Capabilities:\nNone\n\nRemote-control command(s):\n[CONFigure:]DUT:PROFile:SIMSlot<no>:CAPability:IMS"}, {"Level"=4, "Class Only"=TRUE, "Identifier"="", "Descriptive Name"="RF Connections", "Data Type"=0, "Command"="", "Access"=0, "Range Table"="", "Read Callback"="", "Write Callback"="", "Supported Models"="", "Instrument Options"="", "Flags"=0, "Help"="For routing, the system handles RF connections, also called \"signal paths\" in remote control."}, {"Level"=5, "Class Only"=FALSE, "Identifier"="RSCMXPBASE_ATTR_HIDDEN_RF_CONNECTION_ADD", "Descriptive Name"="Hidden RF Connection Add", "Data Type"=6, "Command"="CRE:TENV:SPAT", "Access"=1, "Range Table"="", "Read Callback"="", "Write Callback"="", "Supported Models"="", "Instrument Options"="", "Flags"=8, "Help"="Creates a signal path for a selected connector and assigns a name to the path.\n\nAssign a unique name to each named object within the test environment. Assigning an already used name can be rejected with an error message, even if the other object has not the same type as the new object.\n\nAvailable Repeated Capabilities:\nNone\n\nRemote-control command(s):\nCREate:TENVironment:SPATh"}, {"Level"=5, "Class Only"=FALSE, "Identifier"="RSCMXPBASE_ATTR_RF_CONNECTION_DELETE", "Descriptive Name"="RF Connection Delete", "Data Type"=2, "Command"="DEL:TENV:SPAT", "Access"=1, "Range Table"="", "Read Callback"="", "Write Callback"="", "Supported Models"="", "Instrument Options"="", "Flags"=0, "Help"="Deletes a signal path.\n\nAvailable Repeated Capabilities:\nNone\n\nRemote-control command(s):\nDELete:TENVironment:SPATh"}, {"Level"=5, "Class Only"=FALSE, "Identifier"="RSCMXPBASE_ATTR_RF_CONNECTION_CATALOG", "Descriptive Name"="RF Connection Catalog", "Data Type"=2, "Command"="CAT:TENV:SPAT?", "Access"=0, "Range Table"="", "Read Callback"="", "Write Callback"="", "Supported Models"="", "Instrument Options"="", "Flags"=0, "Help"="Returns all signal path names.\n\nAvailable Repeated Capabilities:\nNone\n\nRemote-control command(s):\nCATalog:TENVironment:SPATh?"}, {"Level"=5, "Class Only"=FALSE, "Identifier"="RSCMXPBASE_ATTR_HIDDEN_RF_CONNECTION_INFORMATION", "Descriptive Name"="Hidden RF Connection Information", "Data Type"=6, "Command"="TENV:SPAT:INFO?", "Access"=0, "Range Table"="", "Read Callback"="", "Write Callback"="", "Supported Models"="", "Instrument Options"="", "Flags"=8, "Help"="Returns information about the specified signal path.\n\nAvailable Repeated Capabilities:\nNone\n\nRemote-control command(s):\n[CONFigure:]TENVironment:SPATh:INFO?"}, {"Level"=5, "Class Only"=FALSE, "Identifier"="RSCMXPBASE_ATTR_HIDDEN_SIGNAL_PATH_DIRECTION", "Descriptive Name"="Hidden Signal Path Direction", "Data Type"=6, "Command"="TENV:SPAT:DIR", "Access"=2, "Range Table"="", "Read Callback"="", "Write Callback"="", "Supported Models"="", "Instrument Options"="", "Flags"=8, "Help"="Defines the direction of a signal path (TX/RX of the instrument).\n\nAvailable Repeated Capabilities:\nNone\n\nRemote-control command(s):\n[CONFigure:]TENVironment:SPATh:DIRection"}, {"Level"=3, "Class Only"=TRUE, "Identifier"="", "Descriptive Name"="Active DUT", "Data Type"=0, "Command"="", "Access"=0, "Range Table"="", "Read Callback"="", "Write Callback"="", "Supported Models"="", "Instrument Options"="", "Flags"=0, "Help"="Configures seetings of active DUT used in the test environment."}, {"Level"=4, "Class Only"=FALSE, "Identifier"="RSCMXPBASE_ATTR_DUT_ACTIVE", "Descriptive Name"="DUT Active", "Data Type"=2, "Command"="SENS:DUT:ACT?", "Access"=0, "Range Table"="", "Read Callback"="", "Write Callback"="", "Supported Models"="", "Instrument Options"="", "Flags"=0, "Help"="Queries the name of the active DUT.\n\nAvailable Repeated Capabilities:\nNone\n\nRemote-control command(s):\nSENSe:DUT:ACTive?"}, {"Level"=4, "Class Only"=FALSE, "Identifier"="RSCMXPBASE_ATTR_DUT_ACTIVATE", "Descriptive Name"="DUT Activate", "Data Type"=2, "Command"="ACT:DUT", "Access"=1, "Range Table"="", "Read Callback"="", "Write Callback"="", "Supported Models"="", "Instrument Options"="", "Flags"=0, "Help"="Activates the DUT with the specified name for usage in the test environment.\n\nAvailable Repeated Capabilities:\nNone\n\nRemote-control command(s):\nACTivate:DUT"}, {"Level"=4, "Class Only"=FALSE, "Identifier"="RSCMXPBASE_ATTR_SELECT_ACTIVE_DUT_SIM_SLOT", "Descriptive Name"="Select Active DUT SIM Slot", "Data Type"=0, "Command"="", "Access"=2, "Range Table"="", "Read Callback"="", "Write Callback"="", "Supported Models"="", "Instrument Options"="", "Flags"=0, "Help"="Selects a SIM slot number for the active DUT.\n\nAvailable Repeated Capabilities:\nNone\n\nRemote-control command(s):\n"}, {"Level"=4, "Class Only"=TRUE, "Identifier"="", "Descriptive Name"="Band Restrictions", "Data Type"=0, "Command"="", "Access"=0, "Range Table"="", "Read Callback"="", "Write Callback"="", "Supported Models"="", "Instrument Options"="", "Flags"=0, "Help"="Downscales the number of used TX and RX DUT connectors for a specific test session."}, {"Level"=5, "Class Only"=FALSE, "Identifier"="RSCMXPBASE_ATTR_ACTIVE_DUT_BAND_RESTRICTIONS_ENABLED", "Descriptive Name"="Active DUT Band Restrictions Enabled", "Data Type"=3, "Command"="DUT:BAND:REST:ENAB", "Access"=2, "Range Table"="", "Read Callback"="", "Write Callback"="", "Supported Models"="", "Instrument Options"="", "Flags"=0, "Help"="Enables restrictions on the number of used DUT connectors for the active DUT.\n\nAvailable Repeated Capabilities:\nNone\n\nRemote-control command(s):\n[CONFigure:]DUT:BAND:RESTrictions:ENABle"}, {"Level"=5, "Class Only"=FALSE, "Identifier"="RSCMXPBASE_ATTR_ACTIVE_DUT_BAND_RESTRICTIONS_CATALOG", "Descriptive Name"="Active DUT Band Restrictions Catalog", "Data Type"=2, "Command"="CAT:DUT:BAND:REST?", "Access"=0, "Range Table"="", "Read Callback"="", "Write Callback"="", "Supported Models"="", "Instrument Options"="", "Flags"=0, "Help"="Queries the DUT connector restrictions for the active DUT.\n\nAvailable Repeated Capabilities:\nNone\n\nRemote-control command(s):\nCATalog:DUT:BAND:RESTrictions?"}, {"Level"=5, "Class Only"=FALSE, "Identifier"="RSCMXPBASE_ATTR_HIDDEN_ACTIVE_DUT_BAND_RESTRICTIONS", "Descriptive Name"="Hidden Active DUT Band Restrictions", "Data Type"=6, "Command"="DUT:BAND:REST", "Access"=2, "Range Table"="", "Read Callback"="", "Write Callback"="", "Supported Models"="", "Instrument Options"="", "Flags"=8, "Help"="Configures restrictions for a frequency band assigned to connectors of the active DUT.\n\nAvailable Repeated Capabilities:\nNone\n\nRemote-control command(s):\n[CONFigure:]DUT:BAND:RESTrictions"}, {"Level"=4, "Class Only"=TRUE, "Identifier"="", "Descriptive Name"="Runtime Parameters", "Data Type"=0, "Command"="", "Access"=0, "Range Table"="", "Read Callback"="", "Write Callback"="", "Supported Models"="", "Instrument Options"="", "Flags"=0, "Help"="Contains functionality to query runtime parameters reported by the active DUT."}, {"Level"=5, "Class Only"=FALSE, "Identifier"="RSCMXPBASE_ATTR_ACTIVE_DUT_IMS_SUPPORT_ENABLED", "Descriptive Name"="Active DUT IMS Support Enabled", "Data Type"=3, "Command"="DUT:SIMS<ActiveDUTSIMSlot>:UEC:IMS", "Access"=2, "Range Table"="", "Read Callback"="rscmxpbase_FormatActiveSIMSlotRepCapBoolean_ReadCallback.vi", "Write Callback"="rscmxpbase_FormatActiveSIMSlotRepCapBoolean_WriteCallback.vi", "Supported Models"="", "Instrument Options"="", "Flags"=0, "Help"="Selects whether the active DUT supports IP multimedia subsystem (IMS) services.\n\nAvailable Repeated Capabilities:\nNone\n\nRemote-control command(s):\n[CONFigure:]DUT:SIMSlot<SimSlotIdx>:UECapability:IMS"}, {"Level"=5, "Class Only"=FALSE, "Identifier"="RSCMXPBASE_ATTR_ACTIVE_DUT_IMS", "Descriptive Name"="Active DUT IMS", "Data Type"=3, "Command"="SENS:DUT:MOD<ActiveDUTSIMSlot>:CAP:REP:IMS?", "Access"=0, "Range Table"="", "Read Callback"="rscmxpbase_FormatActiveSIMSlotRepCapBoolean_ReadCallback.vi", "Write Callback"="rscmxpbase_FormatActiveSIMSlotRepCapBoolean_WriteCallback.vi", "Supported Models"="", "Instrument Options"="", "Flags"=0, "Help"="Queries the reported IMS capabilities of the active DUT.\n\nAvailable Repeated Capabilities:\nNone\n\nRemote-control command(s):\nSENSe:DUT:MODem<ModemIdx>:CAPability:REPorted:IMS?"}, {"Level"=5, "Class Only"=FALSE, "Identifier"="RSCMXPBASE_ATTR_ACTIVE_DUT_IMEI", "Descriptive Name"="Active DUT IMEI", "Data Type"=2, "Command"="SENS:DUT:MOD<ActiveDUTSIMSlot>:CAP:REP:IMEI?", "Access"=0, "Range Table"="", "Read Callback"="rscmxpbase_FormatActiveSIMSlotRepCapString_ReadCallback.vi", "Write Callback"="rscmxpbase_FormatActiveSIMSlotRepCapString_WriteCallback.vi", "Supported Models"="", "Instrument Options"="", "Flags"=0, "Help"="Queries the reported IMEI of the active DUT.\n\nAvailable Repeated Capabilities:\nNone\n\nRemote-control command(s):\nSENSe:DUT:MODem<ModemIdx>:CAPability:REPorted:IMEI?"}, {"Level"=4, "Class Only"=TRUE, "Identifier"="", "Descriptive Name"="SIM Slot", "Data Type"=0, "Command"="", "Access"=0, "Range Table"="", "Read Callback"="", "Write Callback"="", "Supported Models"="", "Instrument Options"="", "Flags"=0, "Help"="Manages the SIM slots of the active DUT. Each SIM slot has an assigned SIM profile."}, {"Level"=5, "Class Only"=FALSE, "Identifier"="RSCMXPBASE_ATTR_ACTIVE_DUT_SIM_SLOT_ADD", "Descriptive Name"="Active DUT SIM Slot Add", "Data Type"=2, "Command"="CRE:DUT:SIMS", "Access"=1, "Range Table"="", "Read Callback"="", "Write Callback"="", "Supported Models"="", "Instrument Options"="", "Flags"=0, "Help"="Adds a SIM slot with the assigned SIM profile name to the active DUT.\n\nAssign a unique name to each named object within the test environment. Assigning an already used name can be rejected with an error message, even if the other object has not the same type as the new object.\n\nAvailable Repeated Capabilities:\nNone\n\nRemote-control command(s):\nCREate:DUT:SIMSlot"}, {"Level"=5, "Class Only"=FALSE, "Identifier"="RSCMXPBASE_ATTR_ACTIVE_DUT_SIM_SLOT_DELETE", "Descriptive Name"="Active DUT SIM Slot Delete", "Data Type"=0, "Command"="DEL:DUT:SIMS", "Access"=1, "Range Table"="", "Read Callback"="", "Write Callback"="", "Supported Models"="", "Instrument Options"="", "Flags"=0, "Help"="Removes the SIM slot with the number  from the active DUT.\n\nAvailable Repeated Capabilities:\nNone\n\nRemote-control command(s):\nDELete:DUT:SIMSlot"}, {"Level"=5, "Class Only"=FALSE, "Identifier"="RSCMXPBASE_ATTR_ACTIVE_DUT_SIM_SLOT_CATALOG", "Descriptive Name"="Active DUT SIM Slot Catalog", "Data Type"=6, "Command"="CAT:DUT:SIMS?", "Access"=0, "Range Table"="", "Read Callback"="", "Write Callback"="", "Supported Models"="", "Instrument Options"="", "Flags"=0, "Help"="Queries all SIM slots of the active DUT. For each SIM slot, the slot number and the name of the referenced profile are returned: {<SimSlotNo>, <SimProfileName>}1, {...}2, ...\n\nAvailable Repeated Capabilities:\nNone\n\nRemote-control command(s):\nCATalog:DUT:SIMSlot?"}, {"Level"=5, "Class Only"=FALSE, "Identifier"="RSCMXPBASE_ATTR_ACTIVE_DUT_SIM_SLOT_PROFILE", "Descriptive Name"="Active DUT SIM Slot Profile", "Data Type"=2, "Command"="DUT:MOD<ActiveDUTSIMSlot>:SIMS:SIMP", "Access"=2, "Range Table"="", "Read Callback"="rscmxpbase_FormatActiveSIMSlotRepCapString_ReadCallback.vi", "Write Callback"="rscmxpbase_FormatActiveSIMSlotRepCapString_WriteCallback.vi", "Supported Models"="", "Instrument Options"="", "Flags"=0, "Help"="Assigns a SIM profile to a SlM slot of the active DUT.\n\nAvailable Repeated Capabilities:\nNone\n\nRemote-control command(s):\n[CONFigure:]DUT:MODem<ModemIdx>:SIMSlot:SIMProfile"}, {"Level"=4, "Class Only"=TRUE, "Identifier"="", "Descriptive Name"="Bands And Connectors", "Data Type"=0, "Command"="", "Access"=0, "Range Table"="", "Read Callback"="", "Write Callback"="", "Supported Models"="", "Instrument Options"="", "Flags"=0, "Help"="Configure the antenna connectors of the active DUT."}, {"Level"=5, "Class Only"=FALSE, "Identifier"="RSCMXPBASE_ATTR_ACTIVE_DUT_CONNECTOR_ADD", "Descriptive Name"="Active DUT Connector Add", "Data Type"=2, "Command"="CRE:DUT:CONN", "Access"=1, "Range Table"="", "Read Callback"="", "Write Callback"="", "Supported Models"="", "Instrument Options"="", "Flags"=0, "Help"="Creates an antenna connector for the active DUT.\n\nAssign a unique name to each named object within the test environment. Assigning an already used name can be rejected with an error message, even if the other object has not the same type as the new object.\n\nAvailable Repeated Capabilities:\nNone\n\nRemote-control command(s):\nCREate:DUT:CONNector"}, {"Level"=5, "Class Only"=FALSE, "Identifier"="RSCMXPBASE_ATTR_ACTIVE_DUT_CONNECTOR_DELETE", "Descriptive Name"="Active DUT Connector Delete", "Data Type"=2, "Command"="DEL:DUT:CONN", "Access"=1, "Range Table"="", "Read Callback"="", "Write Callback"="", "Supported Models"="", "Instrument Options"="", "Flags"=0, "Help"="Deletes an antenna connector of the active DUT.\n\nAvailable Repeated Capabilities:\nNone\n\nRemote-control command(s):\nDELete:DUT:CONNector"}, {"Level"=5, "Class Only"=FALSE, "Identifier"="RSCMXPBASE_ATTR_ACTIVE_DUT_CONNECTOR_CATALOG", "Descriptive Name"="Active DUT Connector Catalog", "Data Type"=2, "Command"="CAT:DUT:CONN?", "Access"=0, "Range Table"="", "Read Callback"="", "Write Callback"="", "Supported Models"="", "Instrument Options"="", "Flags"=0, "Help"="Queries a list of all antenna connectors of the active DUT.\n\nAvailable Repeated Capabilities:\nNone\n\nRemote-control command(s):\nCATalog:DUT:CONNector?"}, {"Level"=5, "Class Only"=FALSE, "Identifier"="RSCMXPBASE_ATTR_HIDDEN_ACTIVE_DUT_CONNECTOR_BAND_ADD", "Descriptive Name"="Hidden Active DUT Connector Band Add", "Data Type"=6, "Command"="ADD:DUT:CONN:BAND", "Access"=1, "Range Table"="", "Read Callback"="", "Write Callback"="", "Supported Models"="", "Instrument Options"="", "Flags"=8, "Help"="Assigns frequency bands to a single antenna connector of the active DUT (connector-centric approach).\n\nYou can assign several bands with a single command. Specify the technology and the band number for each band.\n\nAvailable Repeated Capabilities:\nNone\n\nRemote-control command(s):\nADD:DUT:CONNector:BAND"}, {"Level"=5, "Class Only"=FALSE, "Identifier"="RSCMXPBASE_ATTR_HIDDEN_ACTIVE_DUT_CONNECTOR_BAND_DELETE", "Descriptive Name"="Hidden Active DUT Connector Band Delete", "Data Type"=6, "Command"="REM:DUT:CONN:BAND", "Access"=1, "Range Table"="", "Read Callback"="", "Write Callback"="", "Supported Models"="", "Instrument Options"="", "Flags"=8, "Help"="Removes frequency bands from an antenna connector of the active DUT (connector-centric approach).\n\nYou can remove several bands with a single command. Specify the technology and the band number for each band.\n\nAvailable Repeated Capabilities:\nNone\n\nRemote-control command(s):\nREMove:DUT:CONNector:BAND"}, {"Level"=5, "Class Only"=FALSE, "Identifier"="RSCMXPBASE_ATTR_HIDDEN_ACTIVE_DUT_CONNECTOR_BANDS_CATALOG", "Descriptive Name"="Hidden Active DUT Connector Bands Catalog", "Data Type"=6, "Command"="CAT:DUT:CONN:BAND?", "Access"=0, "Range Table"="", "Read Callback"="", "Write Callback"="", "Supported Models"="", "Instrument Options"="", "Flags"=8, "Help"="Queries a list of all frequency bands assigned to an antenna connector of the active DUT in connector-centric approach.\n\nThe results are returned as groups of values, with <NoOfBands> pairs of <RatType>, <BandNumber> per group:\n\n{<TX>, <RX>, <NoOfBands>, {<RatType>, <BandNumber>,}<NoOfBands> times} ...\n\nAvailable Repeated Capabilities:\nNone\n\nRemote-control command(s):\nCATalog:DUT:CONNector:BAND?"}, {"Level"=5, "Class Only"=FALSE, "Identifier"="RSCMXPBASE_ATTR_HIDDEN_ACTIVE_DUT_BAND_DELETE", "Descriptive Name"="Hidden Active DUT Band Delete", "Data Type"=6, "Command"="REM:DUT:BAND", "Access"=1, "Range Table"="", "Read Callback"="", "Write Callback"="", "Supported Models"="", "Instrument Options"="", "Flags"=8, "Help"="Removes frequency bands from all antenna connectors of the active DUT.\n\nYou can remove several bands with a single command. Specify the technology and the band number for each band.\n\nAvailable Repeated Capabilities:\nNone\n\nRemote-control command(s):\nREMove:DUT:BAND"}, {"Level"=4, "Class Only"=TRUE, "Identifier"="", "Descriptive Name"="Control", "Data Type"=0, "Command"="", "Access"=0, "Range Table"="", "Read Callback"="", "Write Callback"="", "Supported Models"="", "Instrument Options"="", "Flags"=0, "Help"="Configures the control modes of the active DUT."}, {"Level"=5, "Class Only"=FALSE, "Identifier"="RSCMXPBASE_ATTR_ACTIVE_DUT_CONTROL_MODE", "Descriptive Name"="Active DUT Control Mode", "Data Type"=0, "Command"="DUT:CONT:CMOD", "Access"=2, "Range Table"="rsCmxpBase_rngDUTControlMode", "Read Callback"="", "Write Callback"="", "Supported Models"="", "Instrument Options"="", "Flags"=0, "Help"="Selects the DUT control mode.\n\nAvailable Repeated Capabilities:\nNone\n\nRemote-control command(s):\n[CONFigure:]DUT:CONTrol:CMODe"}, {"Level"=5, "Class Only"=FALSE, "Identifier"="RSCMXPBASE_ATTR_ACTIVE_DUT_CONTROL_IP_ENDPOINT", "Descriptive Name"="Active DUT Control IP Endpoint", "Data Type"=2, "Command"="DUT:CONT:AUTO:EXT:IPAD", "Access"=2, "Range Table"="", "Read Callback"="", "Write Callback"="", "Supported Models"="", "Instrument Options"="", "Flags"=0, "Help"="Specifies an IP address and port for communication with the external automation application.\n\nAvailable Repeated Capabilities:\nNone\n\nRemote-control command(s):\n[CONFigure:]DUT:CONTrol:AUTO:EXTernal:IPADdr"}, {"Level"=5, "Class Only"=FALSE, "Identifier"="RSCMXPBASE_ATTR_ACTIVE_DUT_CONTROL_USER_PROMPT_TIMEOUT", "Descriptive Name"="Active DUT Control User Prompt Timeout", "Data Type"=1, "Command"="DUT:CONT:MAN:UPT", "Access"=2, "Range Table"="", "Read Callback"="", "Write Callback"="", "Supported Models"="", "Instrument Options"="", "Flags"=0, "Help"="Specifies the no answer timeout for a DUT action in manual control mode.\n\nAvailable Repeated Capabilities:\nNone\n\nRemote-control command(s):\n[CONFigure:]DUT:CONTrol:MANual:UPTout"}, {"Level"=5, "Class Only"=FALSE, "Identifier"="RSCMXPBASE_ATTR_ACTIVE_DUT_CONTROL_AUTOMATION_FRAMEWORK", "Descriptive Name"="Active DUT Control Automation Framework", "Data Type"=0, "Command"="DUT:CONT:AUTO:FRAM", "Access"=1, "Range Table"="rsCmxpBase_rngDUTControlAutomationFramework", "Read Callback"="", "Write Callback"="", "Supported Models"="", "Instrument Options"="", "Flags"=0, "Help"="Selects the type of automation.\n\nAvailable Repeated Capabilities:\nNone\n\nRemote-control command(s):\n[CONFigure:]DUT:CONTrol:AUTO:FRAMework"}, {"Level"=5, "Class Only"=TRUE, "Identifier"="", "Descriptive Name"="Automation", "Data Type"=0, "Command"="", "Access"=0, "Range Table"="", "Read Callback"="", "Write Callback"="", "Supported Models"="", "Instrument Options"="", "Flags"=0, "Help"="Controls the connection of the active DUT in automation mode."}, {"Level"=6, "Class Only"=FALSE, "Identifier"="RSCMXPBASE_ATTR_ACTIVE_DUT_AIRPLANE_MODE_ENABLED", "Descriptive Name"="Active DUT Airplane Mode Enabled", "Data Type"=3, "Command"="PROC:DUT:CONT:AIRP", "Access"=1, "Range Table"="", "Read Callback"="", "Write Callback"="", "Supported Models"="", "Instrument Options"="", "Flags"=0, "Help"="Switches the airplane mode at the DUT on or off.\n\nAvailable Repeated Capabilities:\nNone\n\nRemote-control command(s):\nPROCedure:DUT:CONTrol:AIRPlane"}, {"Level"=6, "Class Only"=FALSE, "Identifier"="RSCMXPBASE_ATTR_ACTIVE_DUT_AIRPLANE_MODE_ABORT", "Descriptive Name"="Active DUT Airplane Mode Abort", "Data Type"=4, "Command"="ABOR:DUT:CONT:AIRP", "Access"=1, "Range Table"="", "Read Callback"="", "Write Callback"="", "Supported Models"="", "Instrument Options"="", "Flags"=0, "Help"="Cancels switching the airplane mode at the DUT.\n\nAvailable Repeated Capabilities:\nNone\n\nRemote-control command(s):\nABORt:DUT:CONTrol:AIRPlane"}, {"Level"=6, "Class Only"=FALSE, "Identifier"="RSCMXPBASE_ATTR_HIDDEN_ACTIVE_DUT_AIRPLANE_MODE_STATE", "Descriptive Name"="Hidden Active DUT Airplane Mode State", "Data Type"=6, "Command"="FETC:DUT:CONT:AIRP:STAT?", "Access"=0, "Range Table"="", "Read Callback"="", "Write Callback"="", "Supported Models"="", "Instrument Options"="", "Flags"=8, "Help"="Queries the states of airplane mode actions.\n\nAvailable Repeated Capabilities:\nNone\n\nRemote-control command(s):\nFETCh:DUT:CONTrol:AIRPlane:STATe?"}, {"Level"=6, "Class Only"=FALSE, "Identifier"="RSCMXPBASE_ATTR_ACTIVE_DUT_POWER_CYCLE_START", "Descriptive Name"="Active DUT Power Cycle Start", "Data Type"=4, "Command"="PROC:DUT:CONT:PCYC", "Access"=1, "Range Table"="", "Read Callback"="", "Write Callback"="", "Supported Models"="", "Instrument Options"="", "Flags"=0, "Help"="Starts a power cycle at the DUT.\n\nAvailable Repeated Capabilities:\nNone\n\nRemote-control command(s):\nPROCedure:DUT:CONTrol:PCYCle"}, {"Level"=6, "Class Only"=FALSE, "Identifier"="RSCMXPBASE_ATTR_ACTIVE_DUT_POWER_CYCLE_ABORT", "Descriptive Name"="Active DUT Power Cycle Abort", "Data Type"=4, "Command"="ABOR:DUT:CONT:PCYC", "Access"=1, "Range Table"="", "Read Callback"="", "Write Callback"="", "Supported Models"="", "Instrument Options"="", "Flags"=0, "Help"="Cancels the power cycle action at the DUT.\n\nAvailable Repeated Capabilities:\nNone\n\nRemote-control command(s):\nABORt:DUT:CONTrol:PCYCle"}, {"Level"=6, "Class Only"=FALSE, "Identifier"="RSCMXPBASE_ATTR_ACTIVE_DUT_POWER_CYCLE_STATE", "Descriptive Name"="Active DUT Power Cycle State", "Data Type"=0, "Command"="FETC:DUT:CONT:PCYC:STAT?", "Access"=0, "Range Table"="rsCmxpBase_rngDUTPowerCycleState", "Read Callback"="", "Write Callback"="", "Supported Models"="", "Instrument Options"="", "Flags"=0, "Help"="Queries the state of the power cycle at the DUT.\n\nAvailable Repeated Capabilities:\nNone\n\nRemote-control command(s):\nFETCh:DUT:CONTrol:PCYCle:STATe?"}, {"Level"=6, "Class Only"=FALSE, "Identifier"="RSCMXPBASE_ATTR_ACTIVE_DUT_AUDIO_CALL_ABORT_ACTION", "Descriptive Name"="Active DUT Audio Call Abort Action", "Data Type"=0, "Command"="ABOR:DUT:MOD<ActiveDUTSIMSlot>:CONT:CALL:AUD", "Access"=1, "Range Table"="rsCmxpBase_rngActiveDUTMobileAction", "Read Callback"="rscmxpbase_FormatActiveSIMSlotRepCapInt32_ReadCallback.vi", "Write Callback"="rscmxpbase_FormatActiveSIMSlotRepCapInt32_WriteCallback.vi", "Supported Models"="", "Instrument Options"="", "Flags"=0, "Help"="Cancels an audio call action at the DUT.\n\nAvailable Repeated Capabilities:\nNone\n\nRemote-control command(s):\nABORt:DUT:MODem<ModemIdx>:CONTrol:CALL:AUDio"}, {"Level"=6, "Class Only"=FALSE, "Identifier"="RSCMXPBASE_ATTR_ACTIVE_DUT_AUDIO_CALL_PERFORM_ACTION", "Descriptive Name"="Active DUT Audio Call Perform Action", "Data Type"=0, "Command"="PROC:DUT:MOD<ActiveDUTSIMSlot>:CONT:CALL:AUD", "Access"=1, "Range Table"="rsCmxpBase_rngActiveDUTMobileAction", "Read Callback"="rscmxpbase_FormatActiveSIMSlotRepCapInt32_ReadCallback.vi", "Write Callback"="rscmxpbase_FormatActiveSIMSlotRepCapInt32_WriteCallback.vi", "Supported Models"="", "Instrument Options"="", "Flags"=0, "Help"="Controls the audio call connection.\n\nAvailable Repeated Capabilities:\nNone\n\nRemote-control command(s):\nPROCedure:DUT:MODem<ModemIdx>:CONTrol:CALL:AUDio"}, {"Level"=6, "Class Only"=FALSE, "Identifier"="RSCMXPBASE_ATTR_HIDDEN_ACTIVE_DUT_AUDIO_CALL_ACTION_STATE", "Descriptive Name"="Hidden Active DUT Audio Call Action State", "Data Type"=6, "Command"="FETC:DUT:MOD<ActiveDUTSIMSlot>:CONT:CALL:AUD:STAT?", "Access"=0, "Range Table"="", "Read Callback"="rscmxpbase_FormatActiveSIMSlotRepCapRawString_ReadCallback.vi", "Write Callback"="rscmxpbase_FormatActiveSIMSlotRepCapRawString_WriteCallback.vi", "Supported Models"="", "Instrument Options"="", "Flags"=8, "Help"="Queries the states of audio call actions.\n\nAvailable Repeated Capabilities:\nNone\n\nRemote-control command(s):\nFETCh:DUT:MODem<ModemIdx>:CONTrol:CALL:AUDio:STATe?"}, {"Level"=6, "Class Only"=FALSE, "Identifier"="RSCMXPBASE_ATTR_ACTIVE_DUT_VIDEO_CALL_ABORT_ACTION", "Descriptive Name"="Active DUT Video Call Abort Action", "Data Type"=0, "Command"="ABOR:DUT:MOD<ActiveDUTSIMSlot>:CONT:CALL:VID", "Access"=1, "Range Table"="rsCmxpBase_rngActiveDUTMobileAction", "Read Callback"="rscmxpbase_FormatActiveSIMSlotRepCapInt32_ReadCallback.vi", "Write Callback"="rscmxpbase_FormatActiveSIMSlotRepCapInt32_WriteCallback.vi", "Supported Models"="", "Instrument Options"="", "Flags"=0, "Help"="Cancels a video call action at the DUT.\n\nAvailable Repeated Capabilities:\nNone\n\nRemote-control command(s):\nABORt:DUT:MODem<ModemIdx>:CONTrol:CALL:VIDeo"}, {"Level"=6, "Class Only"=FALSE, "Identifier"="RSCMXPBASE_ATTR_ACTIVE_DUT_VIDEO_CALL_PERFORM_ACTION", "Descriptive Name"="Active DUT Video Call Perform Action", "Data Type"=0, "Command"="PROC:DUT:MOD<ActiveDUTSIMSlot>:CONT:CALL:VID", "Access"=1, "Range Table"="rsCmxpBase_rngActiveDUTMobileAction", "Read Callback"="rscmxpbase_FormatActiveSIMSlotRepCapInt32_ReadCallback.vi", "Write Callback"="rscmxpbase_FormatActiveSIMSlotRepCapInt32_WriteCallback.vi", "Supported Models"="", "Instrument Options"="", "Flags"=0, "Help"="Controls the video call connection.\n\nAvailable Repeated Capabilities:\nNone\n\nRemote-control command(s):\nPROCedure:DUT:MODem<ModemIdx>:CONTrol:CALL:VIDeo"}, {"Level"=6, "Class Only"=FALSE, "Identifier"="RSCMXPBASE_ATTR_HIDDEN_ACTIVE_DUT_VIDEO_CALL_STATE", "Descriptive Name"="Hidden Active DUT Video Call State", "Data Type"=6, "Command"="FETC:DUT:MOD<ActiveDUTSIMSlot>:CONT:CALL:VID:STAT?", "Access"=0, "Range Table"="", "Read Callback"="rscmxpbase_FormatActiveSIMSlotRepCapRawString_ReadCallback.vi", "Write Callback"="rscmxpbase_FormatActiveSIMSlotRepCapRawString_WriteCallback.vi", "Supported Models"="", "Instrument Options"="", "Flags"=8, "Help"="Queries the state of video call actions.\n\nAvailable Repeated Capabilities:\nNone\n\nRemote-control command(s):\nFETCh:DUT:MODem<ModemIdx>:CONTrol:CALL:VIDeo:STATe?"}, {"Level"=6, "Class Only"=FALSE, "Identifier"="RSCMXPBASE_ATTR_ACTIVE_DUT_SMS_ABORT", "Descriptive Name"="Active DUT SMS Abort", "Data Type"=4, "Command"="ABOR:DUT:MOD<ActiveDUTSIMSlot>:CONT:SMS", "Access"=1, "Range Table"="", "Read Callback"="", "Write Callback"="rscmxpbase_FormatActiveSIMSlotRepCapEvent_WriteCallback.vi", "Supported Models"="", "Instrument Options"="", "Flags"=0, "Help"="Cancels the sending of an SMS.\n\nAvailable Repeated Capabilities:\nNone\n\nRemote-control command(s):\nABORt:DUT:MODem<ModemIdx>:CONTrol:SMS"}, {"Level"=6, "Class Only"=FALSE, "Identifier"="RSCMXPBASE_ATTR_ACTIVE_DUT_SMS_SEND", "Descriptive Name"="Active DUT SMS Send", "Data Type"=4, "Command"="PROC:DUT:MOD<ActiveDUTSIMSlot>:CONT:SMS", "Access"=1, "Range Table"="", "Read Callback"="", "Write Callback"="rscmxpbase_FormatActiveSIMSlotRepCapEvent_WriteCallback.vi", "Supported Models"="", "Instrument Options"="", "Flags"=0, "Help"="Sends an SMS with default text to a default number.\n\nAvailable Repeated Capabilities:\nNone\n\nRemote-control command(s):\nPROCedure:DUT:MODem<ModemIdx>:CONTrol:SMS"}, {"Level"=6, "Class Only"=FALSE, "Identifier"="RSCMXPBASE_ATTR_ACTIVE_DUT_SMS_STATE", "Descriptive Name"="Active DUT SMS State", "Data Type"=0, "Command"="FETC:DUT:MOD<ActiveDUTSIMSlot>:CONT:SMS:STAT?", "Access"=0, "Range Table"="rsCmxpBase_rngActiveDUTActionState", "Read Callback"="rscmxpbase_FormatActiveSIMSlotRepCapInt32_ReadCallback.vi", "Write Callback"="rscmxpbase_FormatActiveSIMSlotRepCapInt32_WriteCallback.vi", "Supported Models"="", "Instrument Options"="", "Flags"=0, "Help"="Queries the state of an SMS action.\n\nAvailable Repeated Capabilities:\nNone\n\nRemote-control command(s):\nFETCh:DUT:MODem<ModemIdx>:CONTrol:SMS:STATe?"}, {"Level"=2, "Class Only"=TRUE, "Identifier"="", "Descriptive Name"="SIM Profile Settings", "Data Type"=0, "Command"="", "Access"=0, "Range Table"="", "Read Callback"="", "Write Callback"="", "Supported Models"="", "Instrument Options"="", "Flags"=0, "Help"="The following chapters provide detailed reference information on the remote control commands related to SIM profile settings (...:SIMProfile:... commands)."}, {"Level"=3, "Class Only"=FALSE, "Identifier"="RSCMXPBASE_ATTR_SIM_PROFILE_ADD", "Descriptive Name"="SIM Profile Add", "Data Type"=2, "Command"="CRE:SIMP", "Access"=1, "Range Table"="", "Read Callback"="", "Write Callback"="", "Supported Models"="", "Instrument Options"="", "Flags"=0, "Help"="Creates a SIM profile with the specified name.\n\nAssign a unique name to each named object within the test environment. Assigning an already used name can be rejected with an error message, even if the other object has not the same type as the new object.\n\nAvailable Repeated Capabilities:\nNone\n\nRemote-control command(s):\nCREate:SIMProfile"}, {"Level"=3, "Class Only"=FALSE, "Identifier"="RSCMXPBASE_ATTR_SIM_PROFILE_DELETE", "Descriptive Name"="SIM Profile Delete", "Data Type"=2, "Command"="DEL:SIMP", "Access"=1, "Range Table"="", "Read Callback"="", "Write Callback"="", "Supported Models"="", "Instrument Options"="", "Flags"=0, "Help"="Deletes the SIM profile with the specified name.\n\nAvailable Repeated Capabilities:\nNone\n\nRemote-control command(s):\nDELete:SIMProfile"}, {"Level"=3, "Class Only"=FALSE, "Identifier"="RSCMXPBASE_ATTR_HIDDEN_SIM_PROFILE_DUPLICATE", "Descriptive Name"="Hidden SIM Profile Duplicate", "Data Type"=6, "Command"="COPY:SIMP", "Access"=1, "Range Table"="", "Read Callback"="", "Write Callback"="", "Supported Models"="", "Instrument Options"="", "Flags"=8, "Help"="Creates a SIM profile with a new name as a copy of the profile with the specified name.\n\nAvailable Repeated Capabilities:\nNone\n\nRemote-control command(s):\nCOPY:SIMProfile"}, {"Level"=3, "Class Only"=FALSE, "Identifier"="RSCMXPBASE_ATTR_SIM_PROFILE_CATALOG", "Descriptive Name"="SIM Profile Catalog", "Data Type"=2, "Command"="CAT:SIMP?", "Access"=0, "Range Table"="", "Read Callback"="", "Write Callback"="", "Supported Models"="", "Instrument Options"="", "Flags"=0, "Help"="Queries all existing SIM profiles.\n\nAvailable Repeated Capabilities:\nNone\n\nRemote-control command(s):\nCATalog:SIMProfile?"}, {"Level"=3, "Class Only"=TRUE, "Identifier"="", "Descriptive Name"="USIM", "Data Type"=0, "Command"="", "Access"=0, "Range Table"="", "Read Callback"="", "Write Callback"="", "Supported Models"="", "Instrument Options"="", "Flags"=0, "Help"="Configure the USIM parameters of the SIM profile."}, {"Level"=4, "Class Only"=FALSE, "Identifier"="RSCMXPBASE_ATTR_HIDDEN_USIM_SUCI_KEY_PAIR", "Descriptive Name"="Hidden USIM SUCI Key Pair", "Data Type"=6, "Command"="SIMP:USIM:SEC:HNPP", "Access"=2, "Range Table"="", "Read Callback"="", "Write Callback"="", "Supported Models"="", "Instrument Options"="", "Flags"=8, "Help"="Specifies the subscription concealed identifier (SUCI) as a pair of the home network public key identifier and the home network private key. The home network private key is entered as a 64-digit hexadecimal number.\n\nAvailable Repeated Capabilities:\nNone\n\nRemote-control command(s):\n[CONFigure:]SIMProfile:USIM:SECurity:HNPPkpair"}, {"Level"=4, "Class Only"=FALSE, "Identifier"="RSCMXPBASE_ATTR_HIDDEN_USIM_DELETE_SUCI_KEY_PAIR", "Descriptive Name"="Hidden USIM Delete SUCI Key Pair", "Data Type"=6, "Command"="DEL:SIMP:USIM:SEC:HNPP", "Access"=1, "Range Table"="", "Read Callback"="", "Write Callback"="", "Supported Models"="", "Instrument Options"="", "Flags"=8, "Help"="Deletes the home network private key and as a consequence the subscription concealed identifier (SUCI). The home network private key is entered as a 64-digit hexadecimal number.\n\nAvailable Repeated Capabilities:\nNone\n\nRemote-control command(s):\nDELete:SIMProfile:USIM:SECurity:HNPPkpair"}, {"Level"=4, "Class Only"=FALSE, "Identifier"="RSCMXPBASE_ATTR_HIDDEN_USIM_XOR_RES_LENGTH", "Descriptive Name"="Hidden USIM XOR Res Length", "Data Type"=6, "Command"="SIMP:USIM:SEC:XORL", "Access"=2, "Range Table"="", "Read Callback"="", "Write Callback"="", "Supported Models"="", "Instrument Options"="", "Flags"=8, "Help"="Specifies the length of the RES (L2) for XOR authentication algorithms.\n\nAvailable Repeated Capabilities:\nNone\n\nRemote-control command(s):\n[CONFigure:]SIMProfile:USIM:SECurity:XORLength"}, {"Level"=4, "Class Only"=FALSE, "Identifier"="RSCMXPBASE_ATTR_HIDDEN_USIM_SUCI_CATALOG", "Descriptive Name"="Hidden USIM SUCI Catalog", "Data Type"=6, "Command"="CAT:SIMP:USIM:SEC:HNPP?", "Access"=0, "Range Table"="", "Read Callback"="", "Write Callback"="", "Supported Models"="", "Instrument Options"="", "Flags"=8, "Help"="Queries a list of all existing subscription concealed identifiers (SUCIs). For each SUCI, two values are returned:\n\n{<Key>, <PrivateKey>}SUCI 1, {<Key>, <PrivateKey>}SUCI 2, ...\n\nAvailable Repeated Capabilities:\nNone\n\nRemote-control command(s):\nCATalog:SIMProfile:USIM:SECurity:HNPPkpair?"}, {"Level"=4, "Class Only"=FALSE, "Identifier"="RSCMXPBASE_ATTR_USIM_MOBILE_COUNTRY_CODE", "Descriptive Name"="USIM Mobile Country Code", "Data Type"=6, "Command"="SIMP:USIM:MCC", "Access"=1, "Range Table"="", "Read Callback"="", "Write Callback"="", "Supported Models"="", "Instrument Options"="", "Flags"=0, "Help"="Specifies the three-digit mobile country code (MCC).\n\nAvailable Repeated Capabilities:\nNone\n\nRemote-control command(s):\n[CONFigure:]SIMProfile:USIM:MCC"}, {"Level"=4, "Class Only"=FALSE, "Identifier"="RSCMXPBASE_ATTR_HIDDEN_USIM_QUERY_MOBILE_COUNTRY_CODE", "Descriptive Name"="USIM Query Mobile Country Code", "Data Type"=2, "Command"="SIMP:USIM:MCC?", "Access"=0, "Range Table"="", "Read Callback"="", "Write Callback"="", "Supported Models"="", "Instrument Options"="", "Flags"=8, "Help"="Queries the three-digit mobile country code (MCC).\n\nAvailable Repeated Capabilities:\nNone\n\nRemote-control command(s):\n[CONFigure:]SIMProfile:USIM:MCC?"}, {"Level"=4, "Class Only"=FALSE, "Identifier"="RSCMXPBASE_ATTR_USIM_MOBILE_NETWORK_CODE", "Descriptive Name"="USIM Mobile Network Code", "Data Type"=6, "Command"="SIMP:USIM:MNC", "Access"=1, "Range Table"="", "Read Callback"="", "Write Callback"="", "Supported Models"="", "Instrument Options"="", "Flags"=0, "Help"="Specifies the mobile network code (MNC).\n\nAvailable Repeated Capabilities:\nNone\n\nRemote-control command(s):\n[CONFigure:]SIMProfile:USIM:MNC"}, {"Level"=4, "Class Only"=FALSE, "Identifier"="RSCMXPBASE_ATTR_HIDDEN_USIM_QUERY_MOBILE_NETWORK_CODE", "Descriptive Name"="USIM Query Mobile Network Code", "Data Type"=6, "Command"="SIMP:USIM:MNC?", "Access"=0, "Range Table"="", "Read Callback"="", "Write Callback"="", "Supported Models"="", "Instrument Options"="", "Flags"=8, "Help"="Specifies the mobile network code (MNC).\n\nAvailable Repeated Capabilities:\nNone\n\nRemote-control command(s):\n[CONFigure:]SIMProfile:USIM:MNC?"}, {"Level"=4, "Class Only"=FALSE, "Identifier"="RSCMXPBASE_ATTR_USIM_MOBILE_SUBSCRIBER_IDENTIFICATION_NUMBER", "Descriptive Name"="USIM Mobile Subscriber Identification Number", "Data Type"=6, "Command"="SIMP:USIM:MSIN", "Access"=1, "Range Table"="", "Read Callback"="", "Write Callback"="", "Supported Models"="", "Instrument Options"="", "Flags"=0, "Help"="Specifies the mobile subscriber identification number (MSIN).\n\nAvailable Repeated Capabilities:\nNone\n\nRemote-control command(s):\n[CONFigure:]SIMProfile:USIM:MSIN"}, {"Level"=4, "Class Only"=FALSE, "Identifier"="RSCMXPBASE_ATTR_HIDDEN_USIM_QUERY_MOBILE_SUBSCRIBER_IDENTIFICATION_NUMBER", "Descriptive Name"="USIM Query Mobile Subscriber Identification Number", "Data Type"=2, "Command"="SIMP:USIM:MSIN?", "Access"=0, "Range Table"="", "Read Callback"="", "Write Callback"="", "Supported Models"="", "Instrument Options"="", "Flags"=8, "Help"="Queries the mobile subscriber identification number (MSIN).\n\nAvailable Repeated Capabilities:\nNone\n\nRemote-control command(s):\n[CONFigure:]SIMProfile:USIM:MSIN?"}, {"Level"=4, "Class Only"=TRUE, "Identifier"="", "Descriptive Name"="Security", "Data Type"=0, "Command"="", "Access"=0, "Range Table"="", "Read Callback"="", "Write Callback"="", "Supported Models"="", "Instrument Options"="", "Flags"=0, "Help"="Configure the USIM security parameters of the SIM profile"}, {"Level"=5, "Class Only"=FALSE, "Identifier"="RSCMXPBASE_ATTR_USIM_AUTHENTICATION_ALGORITHM", "Descriptive Name"="USIM Authentication Algorithm", "Data Type"=6, "Command"="SIMP:USIM:SEC:AUTH", "Access"=1, "Range Table"="", "Read Callback"="", "Write Callback"="", "Supported Models"="", "Instrument Options"="", "Flags"=0, "Help"="Selects an algorithm for authentication.\n\nAvailable Repeated Capabilities:\nNone\n\nRemote-control command(s):\n[CONFigure:]SIMProfile:USIM:SECurity:AUTHentic"}, {"Level"=5, "Class Only"=FALSE, "Identifier"="RSCMXPBASE_ATTR_HIDDEN_USIM_QUERY_AUTHENTICATION_ALGORITHM", "Descriptive Name"="USIM Query Authentication Algorithm", "Data Type"=0, "Command"="SIMP:USIM:SEC:AUTH?", "Access"=0, "Range Table"="rsCmxpBase_rngAuthenticationAlgorithm", "Read Callback"="", "Write Callback"="", "Supported Models"="", "Instrument Options"="", "Flags"=8, "Help"="Selects an algorithm for authentication.\n\nAvailable Repeated Capabilities:\nNone\n\nRemote-control command(s):\n[CONFigure:]SIMProfile:USIM:SECurity:AUTHentic?"}, {"Level"=5, "Class Only"=FALSE, "Identifier"="RSCMXPBASE_ATTR_USIM_SECRET_KEY", "Descriptive Name"="USIM Secret Key", "Data Type"=6, "Command"="SIMP:USIM:SEC:SKEY", "Access"=1, "Range Table"="", "Read Callback"="", "Write Callback"="", "Supported Models"="", "Instrument Options"="", "Flags"=0, "Help"="Defines the secret key as 32-digit hexadecimal number. The secret key is used for the authentication procedure including a possible integrity check.\n\nAvailable Repeated Capabilities:\nNone\n\nRemote-control command(s):\n[CONFigure:]SIMProfile:USIM:SECurity:SKEY"}, {"Level"=5, "Class Only"=FALSE, "Identifier"="RSCMXPBASE_ATTR_HIDDEN_USIM_QUERY_SECRET_KEY", "Descriptive Name"="USIM Query Secret Key", "Data Type"=6, "Command"="SIMP:USIM:SEC:SKEY?", "Access"=0, "Range Table"="", "Read Callback"="", "Write Callback"="", "Supported Models"="", "Instrument Options"="", "Flags"=8, "Help"="Queries the secret key as 32-digit hexadecimal number. The secret key is used for the authentication procedure including a possible integrity check.\n\nAvailable Repeated Capabilities:\nNone\n\nRemote-control command(s):\n[CONFigure:]SIMProfile:USIM:SECurity:SKEY?"}, {"Level"=5, "Class Only"=FALSE, "Identifier"="RSCMXPBASE_ATTR_USIM_AUTHENTICATION_MANAGEMENT_FIELD", "Descriptive Name"="USIM Authentication Management Field", "Data Type"=6, "Command"="SIMP:USIM:SEC:AMF", "Access"=1, "Range Table"="", "Read Callback"="", "Write Callback"="", "Supported Models"="", "Instrument Options"="", "Flags"=0, "Help"="Specifies the authentication management field (AMF) as four-digit hexadecimal number.\n\nAvailable Repeated Capabilities:\nNone\n\nRemote-control command(s):\n[CONFigure:]SIMProfile:USIM:SECurity:AMField"}, {"Level"=5, "Class Only"=FALSE, "Identifier"="RSCMXPBASE_ATTR_HIDDEN_USIM_QUERY_AUTHENTICATION_MANAGEMENT_FIELD", "Descriptive Name"="USIM Query Authentication Management Field", "Data Type"=2, "Command"="SIMP:USIM:SEC:AMF?", "Access"=0, "Range Table"="", "Read Callback"="", "Write Callback"="", "Supported Models"="", "Instrument Options"="", "Flags"=8, "Help"="Queries the authentication management field (AMF) as four-digit hexadecimal number.\n\nAvailable Repeated Capabilities:\nNone\n\nRemote-control command(s):\n[CONFigure:]SIMProfile:USIM:SECurity:AMField?"}, {"Level"=5, "Class Only"=FALSE, "Identifier"="RSCMXPBASE_ATTR_USIM_OPERATOR_CODE", "Descriptive Name"="USIM Operator Code", "Data Type"=6, "Command"="SIMP:USIM:SEC:OCOD", "Access"=1, "Range Table"="", "Read Callback"="", "Write Callback"="", "Supported Models"="", "Instrument Options"="", "Flags"=0, "Help"="Specifies the operator code value stored on the USIM and whether it is stored on the USIM as ciphered value or as plain text value.\n\nAvailable Repeated Capabilities:\nNone\n\nRemote-control command(s):\n[CONFigure:]SIMProfile:USIM:SECurity:OCODe"}, {"Level"=5, "Class Only"=FALSE, "Identifier"="RSCMXPBASE_ATTR_HIDDEN_USIM_QUERY_OPERATOR_CODE", "Descriptive Name"="USIM Query Operator Code", "Data Type"=6, "Command"="SIMP:USIM:SEC:OCOD?", "Access"=0, "Range Table"="", "Read Callback"="", "Write Callback"="", "Supported Models"="", "Instrument Options"="", "Flags"=8, "Help"="Queries the operator code value stored on the USIM and whether it is stored on the USIM as ciphered value or as plain text value.\n\nAvailable Repeated Capabilities:\nNone\n\nRemote-control command(s):\n[CONFigure:]SIMProfile:USIM:SECurity:OCODe?"}, {"Level"=5, "Class Only"=FALSE, "Identifier"="RSCMXPBASE_ATTR_USIM_INCREMENTS_SEQUENCE_NUMBER_ENABLED", "Descriptive Name"="USIM Increments Sequence Number Enabled", "Data Type"=6, "Command"="SIMP:USIM:SEC:SNIN", "Access"=1, "Range Table"="", "Read Callback"="", "Write Callback"="", "Supported Models"="", "Instrument Options"="", "Flags"=0, "Help"="Enables or disables the sequence number incrementation after every authentication.\n\nAvailable Repeated Capabilities:\nNone\n\nRemote-control command(s):\n[CONFigure:]SIMProfile:USIM:SECurity:SNINcrement"}, {"Level"=5, "Class Only"=FALSE, "Identifier"="RSCMXPBASE_ATTR_HIDDEN_USIM_QUERY_INCREMENTS_SEQUENCE_NUMBER_ENABLED", "Descriptive Name"="USIM Query Increments Sequence Number Enabled", "Data Type"=2, "Command"="SIMP:USIM:SEC:SNIN?", "Access"=0, "Range Table"="", "Read Callback"="", "Write Callback"="", "Supported Models"="", "Instrument Options"="", "Flags"=8, "Help"="Queries the sequence number incrementation after every authentication.\n\nAvailable Repeated Capabilities:\nNone\n\nRemote-control command(s):\n[CONFigure:]SIMProfile:USIM:SECurity:SNINcrement?"}, {"Level"=3, "Class Only"=TRUE, "Identifier"="", "Descriptive Name"="ISIM", "Data Type"=0, "Command"="", "Access"=0, "Range Table"="", "Read Callback"="", "Write Callback"="", "Supported Models"="", "Instrument Options"="", "Flags"=0, "Help"="Configure the ISIM parameters of the SIM profile."}, {"Level"=4, "Class Only"=FALSE, "Identifier"="RSCMXPBASE_ATTR_ISIM_ENABLED", "Descriptive Name"="ISIM Enabled", "Data Type"=6, "Command"="SIMP:ISIM:ENAB", "Access"=1, "Range Table"="", "Read Callback"="", "Write Callback"="", "Supported Models"="", "Instrument Options"="", "Flags"=0, "Help"="Enables or disables ISIM parameters.\n\nAvailable Repeated Capabilities:\nNone\n\nRemote-control command(s):\n[CONFigure:]SIMProfile:ISIM:ENABle"}, {"Level"=4, "Class Only"=FALSE, "Identifier"="RSCMXPBASE_ATTR_HIDDEN_ISIM_QUERY_ENABLED", "Descriptive Name"="ISIM Query Enabled", "Data Type"=2, "Command"="SIMP:ISIM:ENAB?", "Access"=0, "Range Table"="", "Read Callback"="", "Write Callback"="", "Supported Models"="", "Instrument Options"="", "Flags"=8, "Help"="Queries ISIM parameter.\n\nAvailable Repeated Capabilities:\nNone\n\nRemote-control command(s):\n[CONFigure:]SIMProfile:ISIM:ENABle?"}, {"Level"=4, "Class Only"=FALSE, "Identifier"="RSCMXPBASE_ATTR_ISIM_IP_MULTIMEDIA_PRIVATE_IDENTITY", "Descriptive Name"="ISIM IP Multimedia Private Identity", "Data Type"=6, "Command"="SIMP:ISIM:IMPI", "Access"=1, "Range Table"="", "Read Callback"="", "Write Callback"="", "Supported Models"="", "Instrument Options"="", "Flags"=0, "Help"="Specifies the IP multimedia private identity (IMPI).\n\nAvailable Repeated Capabilities:\nNone\n\nRemote-control command(s):\n[CONFigure:]SIMProfile:ISIM:IMPI"}, {"Level"=4, "Class Only"=FALSE, "Identifier"="RSCMXPBASE_ATTR_HIDDEN_ISIM_QUERY_IP_MULTIMEDIA_PRIVATE_IDENTITY", "Descriptive Name"="ISIM Query IP Multimedia Private Identity", "Data Type"=2, "Command"="SIMP:ISIM:IMPI?", "Access"=0, "Range Table"="", "Read Callback"="", "Write Callback"="", "Supported Models"="", "Instrument Options"="", "Flags"=8, "Help"="Specifies the IP multimedia private identity (IMPI).\n\nAvailable Repeated Capabilities:\nNone\n\nRemote-control command(s):\n[CONFigure:]SIMProfile:ISIM:IMPI?"}, {"Level"=4, "Class Only"=FALSE, "Identifier"="RSCMXPBASE_ATTR_ISIM_IP_MULTIMEDIA_PUBLIC_IDENTITIES", "Descriptive Name"="ISIM IP Multimedia Public Identities", "Data Type"=6, "Command"="SIMP:ISIM:IMPU", "Access"=1, "Range Table"="", "Read Callback"="", "Write Callback"="", "Supported Models"="", "Instrument Options"="", "Flags"=0, "Help"="Specifies the IP multimedia public identities (IMPUs)\n\nAvailable Repeated Capabilities:\nNone\n\nRemote-control command(s):\n[CONFigure:]SIMProfile:ISIM:IMPU"}, {"Level"=4, "Class Only"=FALSE, "Identifier"="RSCMXPBASE_ATTR_HIDDEN_ISIM_QUERY_IP_MULTIMEDIA_PUBLIC_IDENTITIES", "Descriptive Name"="ISIM Query IP Multimedia Public Identities", "Data Type"=6, "Command"="SIMP:ISIM:IMPU?", "Access"=0, "Range Table"="", "Read Callback"="", "Write Callback"="", "Supported Models"="", "Instrument Options"="", "Flags"=8, "Help"="Queries  the IP multimedia public identities (IMPUs)\n\nAvailable Repeated Capabilities:\nNone\n\nRemote-control command(s):\n[CONFigure:]SIMProfile:ISIM:IMPU?"}, {"Level"=4, "Class Only"=TRUE, "Identifier"="", "Descriptive Name"="Security", "Data Type"=0, "Command"="", "Access"=0, "Range Table"="", "Read Callback"="", "Write Callback"="", "Supported Models"="", "Instrument Options"="", "Flags"=0, "Help"="Configure the ISIM security parameters of the SIM profile."}, {"Level"=5, "Class Only"=FALSE, "Identifier"="RSCMXPBASE_ATTR_ISIM_AUTHENTICATION_ALGORITHM", "Descriptive Name"="ISIM Authentication Algorithm", "Data Type"=6, "Command"="SIMP:ISIM:SEC:AUTH", "Access"=1, "Range Table"="", "Read Callback"="", "Write Callback"="", "Supported Models"="", "Instrument Options"="", "Flags"=0, "Help"="Selects an algorithm for authentication.\n\nAvailable Repeated Capabilities:\nNone\n\nRemote-control command(s):\n[CONFigure:]SIMProfile:ISIM:SECurity:AUTHentic"}, {"Level"=5, "Class Only"=FALSE, "Identifier"="RSCMXPBASE_ATTR_HIDDEN_ISIM_QUERY_AUTHENTICATION_ALGORITHM", "Descriptive Name"="ISIM Query Authentication Algorithm", "Data Type"=0, "Command"="SIMP:ISIM:SEC:AUTH?", "Access"=0, "Range Table"="rsCmxpBase_rngAuthenticationAlgorithm", "Read Callback"="", "Write Callback"="", "Supported Models"="", "Instrument Options"="", "Flags"=8, "Help"="Selects an algorithm for authentication.\n\nAvailable Repeated Capabilities:\nNone\n\nRemote-control command(s):\n[CONFigure:]SIMProfile:ISIM:SECurity:AUTHentic?"}, {"Level"=5, "Class Only"=FALSE, "Identifier"="RSCMXPBASE_ATTR_ISIM_SECRET_KEY", "Descriptive Name"="ISIM Secret Key", "Data Type"=6, "Command"="SIMP:ISIM:SEC:SKEY", "Access"=1, "Range Table"="", "Read Callback"="", "Write Callback"="", "Supported Models"="", "Instrument Options"="", "Flags"=0, "Help"="Defines the secret key as 32-digit hexadecimal number. The secret key is used for the authentication procedure including a possible integrity check.\n\nAvailable Repeated Capabilities:\nNone\n\nRemote-control command(s):\n[CONFigure:]SIMProfile:ISIM:SECurity:SKEY"}, {"Level"=5, "Class Only"=FALSE, "Identifier"="RSCMXPBASE_ATTR_HIDDEN_ISIM_QUERY_SECRET_KEY", "Descriptive Name"="ISIM Query Secret Key", "Data Type"=6, "Command"="SIMP:ISIM:SEC:SKEY?", "Access"=0, "Range Table"="", "Read Callback"="", "Write Callback"="", "Supported Models"="", "Instrument Options"="", "Flags"=8, "Help"="Defines the secret key as 32-digit hexadecimal number. The secret key is used for the authentication procedure including a possible integrity check.\n\nAvailable Repeated Capabilities:\nNone\n\nRemote-control command(s):\n[CONFigure:]SIMProfile:ISIM:SECurity:SKEY?"}, {"Level"=5, "Class Only"=FALSE, "Identifier"="RSCMXPBASE_ATTR_ISIM_AUTHENTICATION_MANAGEMENT_FIELD", "Descriptive Name"="ISIM Authentication Management Field", "Data Type"=6, "Command"="SIMP:ISIM:SEC:AMF", "Access"=1, "Range Table"="", "Read Callback"="", "Write Callback"="", "Supported Models"="", "Instrument Options"="", "Flags"=0, "Help"="Specifies the authentication management field (AMF) as four-digit hexadecimal number.\n\nAvailable Repeated Capabilities:\nNone\n\nRemote-control command(s):\n[CONFigure:]SIMProfile:ISIM:SECurity:AMField"}, {"Level"=5, "Class Only"=FALSE, "Identifier"="RSCMXPBASE_ATTR_HIDDEN_ISIM_QUERY_AUTHENTICATION_MANAGEMENT_FIELD", "Descriptive Name"="ISIM Query Authentication Management Field", "Data Type"=2, "Command"="SIMP:ISIM:SEC:AMF?", "Access"=0, "Range Table"="", "Read Callback"="", "Write Callback"="", "Supported Models"="", "Instrument Options"="", "Flags"=8, "Help"="Queries the authentication management field (AMF) as four-digit hexadecimal number.\n\nAvailable Repeated Capabilities:\nNone\n\nRemote-control command(s):\n[CONFigure:]SIMProfile:ISIM:SECurity:AMField?"}, {"Level"=5, "Class Only"=FALSE, "Identifier"="RSCMXPBASE_ATTR_ISIM_OPERATOR_CODE", "Descriptive Name"="ISIM Operator Code", "Data Type"=6, "Command"="SIMP:ISIM:SEC:OCOD", "Access"=1, "Range Table"="", "Read Callback"="", "Write Callback"="", "Supported Models"="", "Instrument Options"="", "Flags"=0, "Help"="Specifies the operator code value stored on the USIM and whether it is stored on the USIM as ciphered value or as plain text value.\n\nAvailable Repeated Capabilities:\nNone\n\nRemote-control command(s):\n[CONFigure:]SIMProfile:ISIM:SECurity:OCODe"}, {"Level"=5, "Class Only"=FALSE, "Identifier"="RSCMXPBASE_ATTR_HIDDEN_ISIM_QUERY_OPERATOR_CODE", "Descriptive Name"="ISIM Query Operator Code", "Data Type"=6, "Command"="SIMP:ISIM:SEC:OCOD?", "Access"=0, "Range Table"="", "Read Callback"="", "Write Callback"="", "Supported Models"="", "Instrument Options"="", "Flags"=8, "Help"="Queries the operator code value stored on the USIM and whether it is stored on the USIM as ciphered value or as plain text value.\n\nAvailable Repeated Capabilities:\nNone\n\nRemote-control command(s):\n[CONFigure:]SIMProfile:ISIM:SECurity:OCODe?"}, {"Level"=5, "Class Only"=FALSE, "Identifier"="RSCMXPBASE_ATTR_ISIM_INCREMENTS_SEQUENCE_NUMBER_ENABLED", "Descriptive Name"="ISIM Increments Sequence Number Enabled", "Data Type"=6, "Command"="SIMP:ISIM:SEC:SNIN", "Access"=1, "Range Table"="", "Read Callback"="", "Write Callback"="", "Supported Models"="", "Instrument Options"="", "Flags"=0, "Help"="Enables or disables the sequence number incrementation after every authentication.\n\nAvailable Repeated Capabilities:\nNone\n\nRemote-control command(s):\n[CONFigure:]SIMProfile:ISIM:SECurity:SNINcrement"}, {"Level"=5, "Class Only"=FALSE, "Identifier"="RSCMXPBASE_ATTR_HIDDEN_ISIM_QUERY_INCREMENTS_SEQUENCE_NUMBER_ENABLED", "Descriptive Name"="ISIM Query Increments Sequence Number Enabled", "Data Type"=2, "Command"="SIMP:ISIM:SEC:SNIN?", "Access"=0, "Range Table"="", "Read Callback"="", "Write Callback"="", "Supported Models"="", "Instrument Options"="", "Flags"=8, "Help"="Queries the sequence number incrementation after every authentication.\n\nAvailable Repeated Capabilities:\nNone\n\nRemote-control command(s):\n[CONFigure:]SIMProfile:ISIM:SECurity:SNINcrement?"}, {"Level"=2, "Class Only"=TRUE, "Identifier"="", "Descriptive Name"="Frequency Dependent Attenuation", "Data Type"=0, "Command"="", "Access"=0, "Range Table"="", "Read Callback"="", "Write Callback"="", "Supported Models"="", "Instrument Options"="", "Flags"=0, "Help"="Contains functionality for administration of correction tables for frequency-dependent attenuation."}, {"Level"=3, "Class Only"=FALSE, "Identifier"="RSCMXPBASE_ATTR_CORRECTION_TABLE_CATALOG", "Descriptive Name"="Correction Table Catalog", "Data Type"=2, "Command"="CAT:SYST:ATT:CTAB?", "Access"=0, "Range Table"="", "Read Callback"="", "Write Callback"="", "Supported Models"="", "Instrument Options"="", "Flags"=0, "Help"="Returns the names of all correction tables.\n\nAvailable Repeated Capabilities:\nNone\n\nRemote-control command(s):\nCATalog:SYSTem:ATTenuation:CTABle?"}, {"Level"=3, "Class Only"=FALSE, "Identifier"="RSCMXPBASE_ATTR_HIDDEN_CORRECTION_TABLE_ADD", "Descriptive Name"="Hidden Correction Table Add", "Data Type"=6, "Command"="CRE:SYST:ATT:CTAB", "Access"=1, "Range Table"="", "Read Callback"="", "Write Callback"="", "Supported Models"="", "Instrument Options"="", "Flags"=8, "Help"="Creates a correction table. You can specify one or more parameter pairs <Frequency>, <Attenuation> to add entries to the table.\n\nAvailable Repeated Capabilities:\nNone\n\nRemote-control command(s):\nCREate:SYSTem:ATTenuation:CTABle"}, {"Level"=3, "Class Only"=FALSE, "Identifier"="RSCMXPBASE_ATTR_CORRECTION_TABLE_DELETE_ALL", "Descriptive Name"="Correction Table Delete All", "Data Type"=4, "Command"="DEL:SYST:ATT:CTAB:ALL", "Access"=1, "Range Table"="", "Read Callback"="", "Write Callback"="", "Supported Models"="", "Instrument Options"="", "Flags"=0, "Help"="Deletes all correction tables.\n\nAvailable Repeated Capabilities:\nNone\n\nRemote-control command(s):\nDELete:SYSTem:ATTenuation:CTABle:ALL"}, {"Level"=3, "Class Only"=FALSE, "Identifier"="RSCMXPBASE_ATTR_CORRECTION_TABLE_DELETE", "Descriptive Name"="Correction Table Delete", "Data Type"=2, "Command"="DEL:SYST:ATT:CTAB", "Access"=1, "Range Table"="", "Read Callback"="", "Write Callback"="", "Supported Models"="", "Instrument Options"="", "Flags"=0, "Help"="Deletes a correction table.\n\nAvailable Repeated Capabilities:\nNone\n\nRemote-control command(s):\nDELete:SYSTem:ATTenuation:CTABle"}, {"Level"=3, "Class Only"=FALSE, "Identifier"="RSCMXPBASE_ATTR_HIDDEN_CORRECTION_TABLE_ADD_ENTRY", "Descriptive Name"="Hidden Correction Table Add Entry", "Data Type"=6, "Command"="ADD:SYST:ATT:CTAB", "Access"=1, "Range Table"="", "Read Callback"="", "Write Callback"="", "Supported Models"="", "Instrument Options"="", "Flags"=8, "Help"="Adds entries to an existing correction table. Specify at least one parameter pair <Frequency>, <Attenuation>.\n\nAvailable Repeated Capabilities:\nNone\n\nRemote-control command(s):\nADD:SYSTem:ATTenuation:CTABle"}, {"Level"=3, "Class Only"=FALSE, "Identifier"="RSCMXPBASE_ATTR_HIDDEN_CORRECTION_TABLE_MODIFY_ENTRY", "Descriptive Name"="Hidden Correction Table Modify Entry", "Data Type"=6, "Command"="MOD:SYST:ATT:CTAB", "Access"=1, "Range Table"="", "Read Callback"="", "Write Callback"="", "Supported Models"="", "Instrument Options"="", "Flags"=8, "Help"="Modifies existing entries of a correction table.\n\nSpecify at least one parameter pair <Frequency>, <Attenuation>. Entries with the specified frequencies must already exist. The attenuation values of these entries are overwritten.\n\nAvailable Repeated Capabilities:\nNone\n\nRemote-control command(s):\nMODify:SYSTem:ATTenuation:CTABle"}, {"Level"=3, "Class Only"=FALSE, "Identifier"="RSCMXPBASE_ATTR_HIDDEN_CORRECTION_TABLE_REMOVE_ENTRY", "Descriptive Name"="Hidden Correction Table Remove Entry", "Data Type"=6, "Command"="REM:SYST:ATT:CTAB", "Access"=1, "Range Table"="", "Read Callback"="", "Write Callback"="", "Supported Models"="", "Instrument Options"="", "Flags"=8, "Help"="Removes entries from an existing correction table.\n\nTo remove a single entry, enter the frequency of the entry as <IntervallStart> and omit <IntervallEnd>.\n\nTo remove all entries in a certain frequency range, enter the lower frequency as <IntervallStart> and the upper frequency as <IntervallEnd>.\n\nAvailable Repeated Capabilities:\nNone\n\nRemote-control command(s):\nREMove:SYSTem:ATTenuation:CTABle"}, {"Level"=3, "Class Only"=FALSE, "Identifier"="RSCMXPBASE_ATTR_HIDDEN_CORRECTION_TABLE_ENTRIES", "Descriptive Name"="Hidden Correction Table Entries", "Data Type"=6, "Command"="SYST:ATT:CTAB:INFO?", "Access"=0, "Range Table"="", "Read Callback"="", "Write Callback"="", "Supported Models"="", "Instrument Options"="", "Flags"=8, "Help"="Returns the entries of a correction table as pairs of values:\n\n {<Frequency>, <Attenuation>}1, {<Frequency>, <Attenuation>}2, ...\n\nAvailable Repeated Capabilities:\nNone\n\nRemote-control command(s):\n[CONFigure:]SYSTem:ATTenuation:CTABle:INFO?"}, {"Level"=3, "Class Only"=FALSE, "Identifier"="RSCMXPBASE_ATTR_HIDDEN_CORRECTION_TABLE_ASSIGN_TO_RX", "Descriptive Name"="Hidden Correction Table Assign To RX", "Data Type"=6, "Command"="TENV:SPAT:CTAB:RX", "Access"=2, "Range Table"="", "Read Callback"="", "Write Callback"="", "Supported Models"="", "Instrument Options"="", "Flags"=8, "Help"="Assigns one or more correction tables to the RX direction of a signal path. If there is an existing assignment, it is overwritten.\n\nThe directions refer to the test instrument (RX of the instrument).\n\nAvailable Repeated Capabilities:\nNone\n\nRemote-control command(s):\n[CONFigure:]TENVironment:SPATh:CTABle:RX"}, {"Level"=3, "Class Only"=FALSE, "Identifier"="RSCMXPBASE_ATTR_HIDDEN_CORRECTION_TABLE_ADD_TO_RX", "Descriptive Name"="Hidden Correction Table Add To RX", "Data Type"=6, "Command"="ADD:TENV:SPAT:CTAB:RX", "Access"=1, "Range Table"="", "Read Callback"="", "Write Callback"="", "Supported Models"="", "Instrument Options"="", "Flags"=8, "Help"="Assigns one or more correction tables to the RX direction of a signal path. If there is an existing assignment, the old assignment is kept and the new assignment is added.\n\nAvailable Repeated Capabilities:\nNone\n\nRemote-control command(s):\nADD:TENVironment:SPATh:CTABle:RX"}, {"Level"=3, "Class Only"=FALSE, "Identifier"="RSCMXPBASE_ATTR_HIDDEN_CORRECTION_TABLE_REMOVE_FROM_RX", "Descriptive Name"="Hidden Correction Table Remove From RX", "Data Type"=6, "Command"="REM:TENV:SPAT:CTAB:RX", "Access"=1, "Range Table"="", "Read Callback"="", "Write Callback"="", "Supported Models"="", "Instrument Options"="", "Flags"=8, "Help"="Removes assigned correction tables from the RX direction of a signal path.\n\nAvailable Repeated Capabilities:\nNone\n\nRemote-control command(s):\nREMove:TENVironment:SPATh:CTABle:RX"}, {"Level"=3, "Class Only"=FALSE, "Identifier"="RSCMXPBASE_ATTR_HIDDEN_CORRECTION_TABLE_ASSIGN_TO_TX", "Descriptive Name"="Hidden Correction Table Assign To TX", "Data Type"=6, "Command"="TENV:SPAT:CTAB:TX", "Access"=2, "Range Table"="", "Read Callback"="", "Write Callback"="", "Supported Models"="", "Instrument Options"="", "Flags"=8, "Help"="Assigns one or more correction tables to the TX direction of a signal path. If there is an existing assignment, it is overwritten.\n\nThe directions refer to the test instrument (TX of the instrument).\n\nAvailable Repeated Capabilities:\nNone\n\nRemote-control command(s):\n[CONFigure:]TENVironment:SPATh:CTABle:TX"}, {"Level"=3, "Class Only"=FALSE, "Identifier"="RSCMXPBASE_ATTR_HIDDEN_CORRECTION_TABLE_ADD_TO_TX", "Descriptive Name"="Hidden Correction Table Add To TX", "Data Type"=6, "Command"="ADD:TENV:SPAT:CTAB:TX", "Access"=1, "Range Table"="", "Read Callback"="", "Write Callback"="", "Supported Models"="", "Instrument Options"="", "Flags"=8, "Help"="Assigns one or more correction tables to the TX direction of a signal path. If there is an existing assignment, the old assignment is kept and the new assignment is added.\n\nAvailable Repeated Capabilities:\nNone\n\nRemote-control command(s):\nADD:TENVironment:SPATh:CTABle:TX"}, {"Level"=3, "Class Only"=FALSE, "Identifier"="RSCMXPBASE_ATTR_HIDDEN_CORRECTION_TABLE_REMOVE_FROM_TX", "Descriptive Name"="Hidden Correction Table Remove From TX", "Data Type"=6, "Command"="REM:TENV:SPAT:CTAB:TX", "Access"=1, "Range Table"="", "Read Callback"="", "Write Callback"="", "Supported Models"="", "Instrument Options"="", "Flags"=8, "Help"="Removes assigned correction tables from the TX direction of a signal path.\n\nAvailable Repeated Capabilities:\nNone\n\nRemote-control command(s):\nREMove:TENVironment:SPATh:CTABle:TX"}, {"Level"=2, "Class Only"=TRUE, "Identifier"="", "Descriptive Name"="LAN Setting", "Data Type"=0, "Command"="", "Access"=0, "Range Table"="", "Read Callback"="", "Write Callback"="", "Supported Models"="", "Instrument Options"="", "Flags"=0, "Help"="The following commands configure LAN connection settings."}, {"Level"=3, "Class Only"=FALSE, "Identifier"="RSCMXPBASE_ATTR_QUERY_NETWORK_HOSTNAME", "Descriptive Name"="Query Network Hostname", "Data Type"=2, "Command"="SYST:COMM:NET:HOST?", "Access"=0, "Range Table"="", "Read Callback"="", "Write Callback"="", "Supported Models"="", "Instrument Options"="", "Flags"=0, "Help"="Queries the host name (computer name) of the R&S CMX500. The host name is part of the VISA address string for LAN-based connections.\n\nAvailable Repeated Capabilities:\nNone\n\nRemote-control command(s):\nSYSTem:COMMunicate:NET:HOSTname?"}, {"Level"=3, "Class Only"=FALSE, "Identifier"="RSCMXPBASE_ATTR_CONFIGURE_NETWORK_ADAPTER", "Descriptive Name"="Configure Network Adapter", "Data Type"=2, "Command"="SYST:COMM:NET:ADAP", "Access"=2, "Range Table"="", "Read Callback"="", "Write Callback"="", "Supported Models"="", "Instrument Options"="", "Flags"=0, "Help"="Selects a LAN network adapter for configuration via other SYSTem:COMMunicate:NET:... commands.\n\nAvailable Repeated Capabilities:\nNone\n\nRemote-control command(s):\nSYSTem:COMMunicate:NET:ADAPter"}, {"Level"=3, "Class Only"=FALSE, "Identifier"="RSCMXPBASE_ATTR_CONFIGURE_NETWORK_IP_ADDRESS", "Descriptive Name"="Configure Network IP Address", "Data Type"=2, "Command"="SYST:COMM:NET:IPAD", "Access"=2, "Range Table"="", "Read Callback"="", "Write Callback"="", "Supported Models"="", "Instrument Options"="", "Flags"=0, "Help"="Manually assigns one or more IPv4 addresses to the network adapter. A query returns the currently assigned addresses, irrespective of whether they have been assigned manually or via DHCP.\n\nAvailable Repeated Capabilities:\nNone\n\nRemote-control command(s):\nSYSTem:COMMunicate:NET:IPADdress"}, {"Level"=3, "Class Only"=FALSE, "Identifier"="RSCMXPBASE_ATTR_CONFIGURE_NETWORK_SUBNET_MASK", "Descriptive Name"="Configure Network Subnet Mask", "Data Type"=2, "Command"="SYST:COMM:NET:SUBN:MASK", "Access"=2, "Range Table"="", "Read Callback"="", "Write Callback"="", "Supported Models"="", "Instrument Options"="", "Flags"=0, "Help"="Manually defines the subnet masks to be used for the network adapter IPv4 addresses. A query returns the currently used subnet masks, irrespective of whether they have been assigned manually or via DHCP.\n\nAvailable Repeated Capabilities:\nNone\n\nRemote-control command(s):\nSYSTem:COMMunicate:NET:SUBNet:MASK"}, {"Level"=3, "Class Only"=FALSE, "Identifier"="RSCMXPBASE_ATTR_CONFIGURE_NETWORK_GATEWAY", "Descriptive Name"="Configure Network Gateway", "Data Type"=2, "Command"="SYST:COMM:NET:GAT", "Access"=2, "Range Table"="", "Read Callback"="", "Write Callback"="", "Supported Models"="", "Instrument Options"="", "Flags"=0, "Help"="Manually defines IPv4 addresses of default gateways. A query returns the currently defined addresses, irrespective of whether they have been specified manually or via DHCP.\n\nAvailable Repeated Capabilities:\nNone\n\nRemote-control command(s):\nSYSTem:COMMunicate:NET:GATeway"}, {"Level"=3, "Class Only"=FALSE, "Identifier"="RSCMXPBASE_ATTR_CONFIGURE_NETWORK_DNS", "Descriptive Name"="Configure Network DNS", "Data Type"=2, "Command"="SYST:COMM:NET:DNS", "Access"=2, "Range Table"="", "Read Callback"="", "Write Callback"="", "Supported Models"="", "Instrument Options"="", "Flags"=0, "Help"="Manually defines the DNS server IPv4 addresses to be used. A query returns the defined DNS addresses, irrespective of whether they have been specified manually or via DHCP.\n\nAvailable Repeated Capabilities:\nNone\n\nRemote-control command(s):\nSYSTem:COMMunicate:NET:DNS"}, {"Level"=2, "Class Only"=TRUE, "Identifier"="", "Descriptive Name"="Remote Control Settings", "Data Type"=0, "Command"="", "Access"=0, "Range Table"="", "Read Callback"="", "Write Callback"="", "Supported Models"="", "Instrument Options"="", "Flags"=0, "Help"="The following commands define the address information for the SCPI remote-control interfaces of the R&S CMX500"}, {"Level"=3, "Class Only"=FALSE, "Identifier"="RSCMXPBASE_ATTR_SOCKET_PROTOCOL_MODE", "Descriptive Name"="Socket Protocol Mode", "Data Type"=0, "Command"="SYST:COMM:SOCK{i}:MODE", "Access"=2, "Range Table"="rsCmxpBase_rngProtocolMode", "Read Callback"="", "Write Callback"="", "Supported Models"="", "Instrument Options"="", "Flags"=0, "Help"="Sets the protocol operation mode for direct socket communication.\n\nAvailable Repeated Capabilities:\ni: chan1, chan2, chan3, chan4, chan5, chan6, chan7, chan8, chan9, chan10, chan11, chan12, chan13, chan14, chan15, chan16, chan17, chan18, chan19, chan20, chan21, chan22, chan23, chan24, chan25, chan26, chan27, chan28, chan29, chan30, chan31, chan32\r\n\nRemote-control command(s):\nSYSTem:COMMunicate:SOCKet<i>:MODE"}, {"Level"=3, "Class Only"=FALSE, "Identifier"="RSCMXPBASE_ATTR_SET_DIRECT_PORT_NUMBER", "Descriptive Name"="Set Direct Port Number", "Data Type"=0, "Command"="SYST:COMM:SOCK{i}:PORT", "Access"=2, "Range Table"="rsCmxpBase_rngPortNumber", "Read Callback"="", "Write Callback"="", "Supported Models"="", "Instrument Options"="", "Flags"=0, "Help"="Sets the data port number for direct socket communication.\n\nAvailable Repeated Capabilities:\ni: chan1, chan2, chan3, chan4, chan5, chan6, chan7, chan8, chan9, chan10, chan11, chan12, chan13, chan14, chan15, chan16, chan17, chan18, chan19, chan20, chan21, chan22, chan23, chan24, chan25, chan26, chan27, chan28, chan29, chan30, chan31, chan32\r\n\nRemote-control command(s):\nSYSTem:COMMunicate:SOCKet<i>:PORT"}, {"Level"=3, "Class Only"=FALSE, "Identifier"="RSCMXPBASE_ATTR_SOCKET_VISA_RESOURCE", "Descriptive Name"="Socket VISA Resource", "Data Type"=2, "Command"="SYST:COMM:SOCK{i}:VRES?", "Access"=0, "Range Table"="", "Read Callback"="", "Write Callback"="", "Supported Models"="", "Instrument Options"="", "Flags"=0, "Help"="Queries the VISA resource string for direct socket communication.\n\nAvailable Repeated Capabilities:\ni: chan1, chan2, chan3, chan4, chan5, chan6, chan7, chan8, chan9, chan10, chan11, chan12, chan13, chan14, chan15, chan16, chan17, chan18, chan19, chan20, chan21, chan22, chan23, chan24, chan25, chan26, chan27, chan28, chan29, chan30, chan31, chan32\r\n\nRemote-control command(s):\nSYSTem:COMMunicate:SOCKet<i>:VRESource?"}, {"Level"=3, "Class Only"=FALSE, "Identifier"="RSCMXPBASE_ATTR_USB_VISA_RESOURCE", "Descriptive Name"="USB VISA Resource", "Data Type"=2, "Command"="SYST:COMM:USB:VRES?", "Access"=0, "Range Table"="", "Read Callback"="", "Write Callback"="", "Supported Models"="", "Instrument Options"="", "Flags"=0, "Help"="Queries the VISA resource string of the USB interface.\n\nAvailable Repeated Capabilities:\nNone\n\nRemote-control command(s):\nSYSTem:COMMunicate:USB:VRESource?"}, {"Level"=3, "Class Only"=FALSE, "Identifier"="RSCMXPBASE_ATTR_HISLIP_VISA_RESOURCE", "Descriptive Name"="HiSLIP VISA Resource", "Data Type"=2, "Command"="SYST:COMM:HISL{i}:VRES?", "Access"=0, "Range Table"="", "Read Callback"="", "Write Callback"="", "Supported Models"="", "Instrument Options"="", "Flags"=0, "Help"="Queries the VISA resource string for the HiSLIP protocol.\n\nAvailable Repeated Capabilities:\ni: chan1, chan2, chan3, chan4, chan5, chan6, chan7, chan8, chan9, chan10, chan11, chan12, chan13, chan14, chan15, chan16, chan17, chan18, chan19, chan20, chan21, chan22, chan23, chan24, chan25, chan26, chan27, chan28, chan29, chan30, chan31, chan32\r\n\nRemote-control command(s):\nSYSTem:COMMunicate:HISLip<i>:VRESource?"}, {"Level"=3, "Class Only"=FALSE, "Identifier"="RSCMXPBASE_ATTR_ENABLE_VXI11_INTERFACE", "Descriptive Name"="Enable VXI-11 Interface", "Data Type"=3, "Command"="SYST:COMM:VXI{i}:GTR", "Access"=2, "Range Table"="", "Read Callback"="", "Write Callback"="", "Supported Models"="", "Instrument Options"="", "Flags"=0, "Help"="Enables or disables the VXI-11 interface.\n\nAvailable Repeated Capabilities:\ni: chan1, chan2, chan3, chan4, chan5, chan6, chan7, chan8, chan9, chan10, chan11, chan12, chan13, chan14, chan15, chan16, chan17, chan18, chan19, chan20, chan21, chan22, chan23, chan24, chan25, chan26, chan27, chan28, chan29, chan30, chan31, chan32\r\n\nRemote-control command(s):\nSYSTem:COMMunicate:VXI<i>:GTR"}, {"Level"=3, "Class Only"=FALSE, "Identifier"="RSCMXPBASE_ATTR_VXI11_VISA_RESOURCE", "Descriptive Name"="VXI-11 VISA Resource", "Data Type"=2, "Command"="SYST:COMM:VXI{i}:VRES?", "Access"=0, "Range Table"="", "Read Callback"="", "Write Callback"="", "Supported Models"="", "Instrument Options"="", "Flags"=0, "Help"="Queries the VISA resource string for the VXI-11 protocol.\n\nAvailable Repeated Capabilities:\ni: chan1, chan2, chan3, chan4, chan5, chan6, chan7, chan8, chan9, chan10, chan11, chan12, chan13, chan14, chan15, chan16, chan17, chan18, chan19, chan20, chan21, chan22, chan23, chan24, chan25, chan26, chan27, chan28, chan29, chan30, chan31, chan32\r\n\nRemote-control command(s):\nSYSTem:COMMunicate:VXI<i>:VRESource?"}, {"Level"=2, "Class Only"=TRUE, "Identifier"="", "Descriptive Name"="Remote Trace", "Data Type"=0, "Command"="", "Access"=0, "Range Table"="", "Read Callback"="", "Write Callback"="", "Supported Models"="", "Instrument Options"="", "Flags"=0, "Help"="Contains functionality for monitoring the remote control interface."}, {"Level"=3, "Class Only"=FALSE, "Identifier"="RSCMXPBASE_ATTR_REMOTE_TRACE_ACTIVE", "Descriptive Name"="Remote Trace Active", "Data Type"=3, "Command"="BASE:RTR:ACT", "Access"=2, "Range Table"="", "Read Callback"="", "Write Callback"="", "Supported Models"="", "Instrument Options"="", "Flags"=0, "Help"="Enables tracing.\n\nAvailable Repeated Capabilities:\nNone\n\nRemote-control command(s):\n[CONFigure:]BASE:RTRace:ACTive"}, {"Level"=3, "Class Only"=FALSE, "Identifier"="RSCMXPBASE_ATTR_REMOTE_TRACE_AUTOSCROLL_ENABLED", "Descriptive Name"="Remote Trace Autoscroll Enabled", "Data Type"=3, "Command"="BASE:RTR:ASCR", "Access"=2, "Range Table"="", "Read Callback"="", "Write Callback"="", "Supported Models"="", "Instrument Options"="", "Flags"=0, "Help"="Enables automatic scrolling for the trace log on the screen.\n\nAvailable Repeated Capabilities:\nNone\n\nRemote-control command(s):\n[CONFigure:]BASE:RTRace:ASCRoll"}, {"Level"=3, "Class Only"=FALSE, "Identifier"="RSCMXPBASE_ATTR_HIDDEN_REMOTE_TRACE_DESTINATION", "Descriptive Name"="Hidden Remote Trace Destination", "Data Type"=6, "Command"="BASE:RTR:TARG", "Access"=2, "Range Table"="", "Read Callback"="", "Write Callback"="", "Supported Models"="", "Instrument Options"="", "Flags"=8, "Help"="Selects the trace log destination. You can display the log in the GUI and/or write the results to a file.\n\nAvailable Repeated Capabilities:\nNone\n\nRemote-control command(s):\n[CONFigure:]BASE:RTRace:TARGet"}, {"Level"=3, "Class Only"=FALSE, "Identifier"="RSCMXPBASE_ATTR_REMOTE_TRACE_CLEAR", "Descriptive Name"="Remote Trace Clear", "Data Type"=4, "Command"="BASE:RTR:CLE", "Access"=1, "Range Table"="", "Read Callback"="", "Write Callback"="", "Supported Models"="", "Instrument Options"="", "Flags"=0, "Help"="Resets the numbering of the trace log rows. The next entry gets the ID 1.\n\nAvailable Repeated Capabilities:\nNone\n\nRemote-control command(s):\n[CONFigure:]BASE:RTRace:CLEar"}, {"Level"=3, "Class Only"=FALSE, "Identifier"="RSCMXPBASE_ATTR_REMOTE_TRACE_CONNECTION_ACTIVE", "Descriptive Name"="Remote Trace Connection Active", "Data Type"=3, "Command"="BASE:RTR:CLIS:ACT", "Access"=2, "Range Table"="", "Read Callback"="", "Write Callback"="", "Supported Models"="", "Instrument Options"="", "Flags"=0, "Help"="Enables the connection list (contents that can be queried via RSCMXPBASE_ATTR_REMOTE_TRACE_CONNECTION_LIST_SECTION).\n\nAvailable Repeated Capabilities:\nNone\n\nRemote-control command(s):\n[CONFigure:]BASE:RTRace:CLISt:ACTive"}, {"Level"=3, "Class Only"=FALSE, "Identifier"="RSCMXPBASE_ATTR_HIDDEN_REMOTE_TRACE_CONNECTION_COUNT", "Descriptive Name"="Hidden Remote Trace Connection Count", "Data Type"=6, "Command"="FETC:BASE:RTR:CONN:COUN?", "Access"=0, "Range Table"="", "Read Callback"="", "Write Callback"="", "Supported Models"="", "Instrument Options"="", "Flags"=8, "Help"="Queries the number of remote control connections.\n\nAvailable Repeated Capabilities:\nNone\n\nRemote-control command(s):\nFETCh:BASE:RTRace:CONNections:COUNt?"}, {"Level"=3, "Class Only"=FALSE, "Identifier"="RSCMXPBASE_ATTR_REMOTE_TRACE_CONNECTION_LIST_SECTION", "Descriptive Name"="Remote Trace Connection List Section", "Data Type"=6, "Command"="FETC:BASE:RTR:CONN:ROWS?", "Access"=0, "Range Table"="", "Read Callback"="", "Write Callback"="", "Supported Models"="", "Instrument Options"="", "Flags"=0, "Help"="Queries the contents of the connection list. There is one set of results per connection:\n\n{<ConnectionId>, <TestEnvironment>, <TimeStamp>, <VisaResource>, <ConnectionType>}conn 1, {...}conn 2, {...}conn 3, ...\n\nAvailable Repeated Capabilities:\nNone\n\nRemote-control command(s):\nFETCh:BASE:RTRace:CONNection:ROWS?"}, {"Level"=3, "Class Only"=FALSE, "Identifier"="RSCMXPBASE_ATTR_REMOTE_TRACE_HEADER_FILTER_SECTION", "Descriptive Name"="Remote Trace Header Filter Section", "Data Type"=0, "Command"="BASE:RTR:COL", "Access"=2, "Range Table"="rsCmxpBase_rngRemoteTraceHeaderFilter", "Read Callback"="", "Write Callback"="", "Supported Models"="", "Instrument Options"="", "Flags"=0, "Help"="Selects which columns are shown in the trace log on the screen.\n\nAvailable Repeated Capabilities:\nNone\n\nRemote-control command(s):\n[CONFigure:]BASE:RTRace:COLumns"}, {"Level"=3, "Class Only"=FALSE, "Identifier"="RSCMXPBASE_ATTR_HIDDEN_REMOTE_TRACE_EVENTS", "Descriptive Name"="Hidden Remote Trace Events", "Data Type"=6, "Command"="BASE:RTR:EVEN", "Access"=2, "Range Table"="", "Read Callback"="", "Write Callback"="", "Supported Models"="", "Instrument Options"="", "Flags"=8, "Help"="Selects which types of events are reported in the trace log.\n\nAvailable Repeated Capabilities:\nNone\n\nRemote-control command(s):\n[CONFigure:]BASE:RTRace:EVENts"}, {"Level"=3, "Class Only"=FALSE, "Identifier"="RSCMXPBASE_ATTR_REMOTE_TRACE_LOG_CONTENTS", "Descriptive Name"="Remote Trace Log Contents", "Data Type"=2, "Command"="FETC:BASE:RTR:ROWS?", "Access"=0, "Range Table"="", "Read Callback"="", "Write Callback"="", "Supported Models"="", "Instrument Options"="", "Flags"=0, "Help"="Queries the contents of the remote trace log.\n\nAvailable Repeated Capabilities:\nNone\n\nRemote-control command(s):\nFETCh:BASE:RTRace:ROWS?"}, {"Level"=2, "Class Only"=TRUE, "Identifier"="", "Descriptive Name"="Self-Alignment", "Data Type"=0, "Command"="", "Access"=0, "Range Table"="", "Read Callback"="", "Write Callback"="", "Supported Models"="", "Instrument Options"="", "Flags"=0, "Help"="The following commands initiate a self-alignment procedure and query the related status information."}, {"Level"=3, "Class Only"=FALSE, "Identifier"="RSCMXPBASE_ATTR_MEASURMENT_START", "Descriptive Name"="Measurment Start", "Data Type"=4, "Command"="INIT:BASE:SAL", "Access"=1, "Range Table"="", "Read Callback"="", "Write Callback"="", "Supported Models"="", "Instrument Options"="", "Flags"=0, "Help"="Starts the measurement procedure.\n\nAvailable Repeated Capabilities:\nNone\n\nRemote-control command(s):\nINITiate:BASE:SALignment"}, {"Level"=3, "Class Only"=FALSE, "Identifier"="RSCMXPBASE_ATTR_MEASURMENT_STOP", "Descriptive Name"="Measurment Stop", "Data Type"=4, "Command"="STOP:BASE:SAL", "Access"=1, "Range Table"="", "Read Callback"="", "Write Callback"="", "Supported Models"="", "Instrument Options"="", "Flags"=0, "Help"="Pauses the measurement procedure.\n\nAvailable Repeated Capabilities:\nNone\n\nRemote-control command(s):\nSTOP:BASE:SALignment"}, {"Level"=3, "Class Only"=FALSE, "Identifier"="RSCMXPBASE_ATTR_MEASURMENT_ABORT", "Descriptive Name"="Measurment Abort", "Data Type"=4, "Command"="ABOR:BASE:SAL", "Access"=1, "Range Table"="", "Read Callback"="", "Write Callback"="", "Supported Models"="", "Instrument Options"="", "Flags"=0, "Help"="Aborts the measurement procedure.\n\nAvailable Repeated Capabilities:\nNone\n\nRemote-control command(s):\nABORt:BASE:SALignment"}, {"Level"=3, "Class Only"=FALSE, "Identifier"="RSCMXPBASE_ATTR_QUERY_MEASUREMENT_STATE", "Descriptive Name"="Query Measurement State", "Data Type"=0, "Command"="FETC:BASE:SAL?", "Access"=0, "Range Table"="rsCmxpBase_rngQueryMeasurementState", "Read Callback"="", "Write Callback"="", "Supported Models"="", "Instrument Options"="", "Flags"=0, "Help"="Queries the state of the measurement procedure.\n\nAvailable Repeated Capabilities:\nNone\n\nRemote-control command(s):\nFETCh:BASE:SALignment?"}, {"Level"=3, "Class Only"=FALSE, "Identifier"="RSCMXPBASE_ATTR_MEASUREMENT_MODE", "Descriptive Name"="Measurement Mode", "Data Type"=0, "Command"="CONF:BASE:SAL:MODE", "Access"=2, "Range Table"="rsCmxpBase_rngMeasurementMode", "Read Callback"="", "Write Callback"="", "Supported Models"="", "Instrument Options"="", "Flags"=0, "Help"="Selects the measurement mode for self-alignment.\n\nAvailable Repeated Capabilities:\nNone\n\nRemote-control command(s):\nCONFigure:BASE:SALignment:MODE"}, {"Level"=3, "Class Only"=FALSE, "Identifier"="RSCMXPBASE_ATTR_QUERY_LAST_MEASURMENT_MODE", "Descriptive Name"="Query Last Measurment Mode", "Data Type"=6, "Command"="FETC:BASE:SAL:STAT?", "Access"=0, "Range Table"="", "Read Callback"="", "Write Callback"="", "Supported Models"="", "Instrument Options"="", "Flags"=0, "Help"="Queries status information for the last self-alignment execution. The information is returned for the measurement modes 'IQ' or 'Verify IQ' (whichever was executed last) and 'Level': <State>IQ or verify IQ, <State>level\n\nAvailable Repeated Capabilities:\nNone\n\nRemote-control command(s):\nFETCh:BASE:SALignment:STATe?"}, {"Level"=3, "Class Only"=FALSE, "Identifier"="RSCMXPBASE_ATTR_QUERY_LAST_SUCCESFULL_PROCEDURE", "Descriptive Name"="Query Last Succesfull Procedure", "Data Type"=2, "Command"="FETC:BASE:SAL:LVAL?", "Access"=0, "Range Table"="", "Read Callback"="", "Write Callback"="", "Supported Models"="", "Instrument Options"="", "Flags"=0, "Help"="Queries the date and time of the last successful execution of the self-alignment procedure. The information is returned for the measurement modes 'IQ' and 'Level': <Date>IQ, <Time>IQ, <Date>level, <Time>level\n\nAvailable Repeated Capabilities:\nNone\n\nRemote-control command(s):\nFETCh:BASE:SALignment:LVALid?"}, {"Level"=2, "Class Only"=TRUE, "Identifier"="", "Descriptive Name"="Reference Frequency Settings", "Data Type"=0, "Command"="", "Access"=0, "Range Table"="", "Read Callback"="", "Write Callback"="", "Supported Models"="", "Instrument Options"="", "Flags"=0, "Help"="The following commands configure the reference frequency settings."}, {"Level"=3, "Class Only"=FALSE, "Identifier"="RSCMXPBASE_ATTR_SYSTEM_REFERENCE_FREQUENCY_SOURCE", "Descriptive Name"="System Reference Frequency Source", "Data Type"=0, "Command"="SYST:BASE:REF:FREQ:SOUR", "Access"=2, "Range Table"="rsCmxpBase_rngSelectFrequencyFormat", "Read Callback"="", "Write Callback"="", "Supported Models"="", "Instrument Options"="", "Flags"=0, "Help"="Selects the reference frequency source to be used.\n\nAvailable Repeated Capabilities:\nNone\n\nRemote-control command(s):\nSYSTem:BASE:REFerence:FREQuency:SOURce"}, {"Level"=3, "Class Only"=FALSE, "Identifier"="RSCMXPBASE_ATTR_SYSTEM_REFERENCE_EXTERNAL_FREQUENCY", "Descriptive Name"="System Reference External Frequency", "Data Type"=1, "Command"="SYST:BASE:REF:FREQ", "Access"=2, "Range Table"="rsCmxpBase_rngReferenceFrequencySettings", "Read Callback"="", "Write Callback"="", "Supported Models"="", "Instrument Options"="", "Flags"=0, "Help"="Sets the R&S CMX500 external reference frequency.\n\nAvailable Repeated Capabilities:\nNone\n\nRemote-control command(s):\nSYSTem:BASE:REFerence:FREQuency"}, {"Level"=3, "Class Only"=FALSE, "Identifier"="RSCMXPBASE_ATTR_REFERENCE_FREQUENCY_STATE", "Descriptive Name"="Reference Frequency State", "Data Type"=3, "Command"="SENS:BASE:REF:FREQ:LOCK?", "Access"=0, "Range Table"="", "Read Callback"="", "Write Callback"="", "Supported Models"="", "Instrument Options"="", "Flags"=0, "Help"="Queries whether the reference frequency is locked or not.\n\nAvailable Repeated Capabilities:\nNone\n\nRemote-control command(s):\nSENSe:BASE:REFerence:FREQuency:LOCKed?"}, {"Level"=2, "Class Only"=TRUE, "Identifier"="", "Descriptive Name"="Trigger", "Data Type"=0, "Command"="", "Access"=0, "Range Table"="", "Read Callback"="", "Write Callback"="", "Supported Models"="", "Instrument Options"="", "Flags"=0, "Help"="Configures the trigger connectors Trig A to Trig E on the rear panel."}, {"Level"=3, "Class Only"=FALSE, "Identifier"="RSCMXPBASE_ATTR_SELECT_TRIGGER", "Descriptive Name"="Select Trigger", "Data Type"=0, "Command"="", "Access"=2, "Range Table"="", "Read Callback"="", "Write Callback"="", "Supported Models"="", "Instrument Options"="", "Flags"=0, "Help"="Selects the instrument suffix. Use RSCMXPBASE_ATTR_TRIGGER_CONNECTOR_CATALOG to query an overview of the instruments and their trigger connectors. The R&S CMX500 is the primary instrument and has the suffix 1.\n\nFor setups with a single instrument, you can omit the suffix.\n\nAvailable Repeated Capabilities:\nNone\n\nRemote-control command(s):\n"}, {"Level"=3, "Class Only"=FALSE, "Identifier"="RSCMXPBASE_ATTR_TRIGGER_CONNECTOR_CATALOG", "Descriptive Name"="Trigger Connector Catalog", "Data Type"=2, "Command"="TRIG:BASE:EXT:CAT?", "Access"=0, "Range Table"="", "Read Callback"="", "Write Callback"="", "Supported Models"="", "Instrument Options"="", "Flags"=0, "Help"="Lists all trigger connectors of the primary instrument and of all instruments controlled by the primary instrument.\n\nIn a multi-box setup, a number <n> is returned for the styles NAME and FQName. The number <n> identifies the instrument. If this command returns an <n> = 0, 1, ... then add 1 to get the value for the suffix <n> in the other commands (1, 2, ...).\n\nFor a single-box setup, the number <n> is omitted in the returned strings and you can omit the suffix <n> in the other commands.\n\nAvailable Repeated Capabilities:\nNone\n\nRemote-control command(s):\nTRIGger:BASE:EXTernal:CATalog?"}, {"Level"=3, "Class Only"=FALSE, "Identifier"="RSCMXPBASE_ATTR_TRIGGER_GENERATE_SIGNAL", "Descriptive Name"="Trigger Generate Signal", "Data Type"=4, "Command"="TRIG:BASE:UIN:EXEC", "Access"=1, "Range Table"="", "Read Callback"="", "Write Callback"="", "Supported Models"="", "Instrument Options"="", "Flags"=0, "Help"="Initiates the generation of a User Initiated Trigger signal.\n\nAvailable Repeated Capabilities:\nNone\n\nRemote-control command(s):\nTRIGger:BASE:UINitiated:EXECute"}, {"Level"=3, "Class Only"=FALSE, "Identifier"="RSCMXPBASE_ATTR_TRIGGER_A_SOURCE_CATALOG", "Descriptive Name"="Trigger A Source Catalog", "Data Type"=2, "Command"="TRIG:BASE:EXTA<Trigger>:CAT:SOUR?", "Access"=0, "Range Table"="", "Read Callback"="rscmxpbase_FormatTriggerRepCapString_ReadCallback.vi", "Write Callback"="rscmxpbase_FormatTriggerRepCapString_WriteCallback.vi", "Supported Models"="", "Instrument Options"="", "Flags"=0, "Help"="Lists all trigger source values that can be set using RSCMXPBASE_ATTR_TRIGGER_A_SOURCE.\n\nAvailable Repeated Capabilities:\nNone\n\nRemote-control command(s):\nTRIGger:BASE:EXTA<n>:CATalog:SOURce?"}, {"Level"=3, "Class Only"=FALSE, "Identifier"="RSCMXPBASE_ATTR_TRIGGER_A_SOURCE", "Descriptive Name"="Trigger A Source", "Data Type"=2, "Command"="TRIG:BASE:EXTA<Trigger>:SOUR", "Access"=2, "Range Table"="", "Read Callback"="rscmxpbase_FormatTriggerRepCapString_ReadCallback.vi", "Write Callback"="rscmxpbase_FormatTriggerRepCapString_WriteCallback.vi", "Supported Models"="", "Instrument Options"="", "Flags"=0, "Help"="Selects the output trigger signals to be routed to the trigger connectors. A list of all supported values can be retrieved using RSCMXPBASE_ATTR_TRIGGER_A_SOURCE_CATALOG.\n\nAvailable Repeated Capabilities:\nNone\n\nRemote-control command(s):\nTRIGger:BASE:EXTA<n>:SOURce"}, {"Level"=3, "Class Only"=FALSE, "Identifier"="RSCMXPBASE_ATTR_TRIGGER_A_DIRECTION", "Descriptive Name"="Trigger A Direction", "Data Type"=0, "Command"="TRIG:BASE:EXTA<Trigger>:DIR", "Access"=2, "Range Table"="rsCmxpBase_rngTriggerDirection", "Read Callback"="rscmxpbase_FormatTriggerRepCapInt32_ReadCallback.vi", "Write Callback"="rscmxpbase_FormatTriggerRepCapInt32_WriteCallback.vi", "Supported Models"="", "Instrument Options"="", "Flags"=0, "Help"="Configures the trigger connectors of an R&SCMW as input or output connectors.\n\nAvailable Repeated Capabilities:\nNone\n\nRemote-control command(s):\nTRIGger:BASE:EXTA<n>:DIRection"}, {"Level"=3, "Class Only"=FALSE, "Identifier"="RSCMXPBASE_ATTR_TRIGGER_A_SLOPE", "Descriptive Name"="Trigger A Slope", "Data Type"=0, "Command"="TRIG:BASE:EXTA<Trigger>:SLOP", "Access"=2, "Range Table"="rsCmxpBase_rngTriggerSlope", "Read Callback"="rscmxpbase_FormatTriggerRepCapInt32_ReadCallback.vi", "Write Callback"="rscmxpbase_FormatTriggerRepCapInt32_WriteCallback.vi", "Supported Models"="", "Instrument Options"="", "Flags"=0, "Help"="Specifies whether the rising edge or the falling edge of the trigger pulse is generated at the trigger event.\n\nThe setting applies to output trigger signals provided at the trigger connectors.\n\nAvailable Repeated Capabilities:\nNone\n\nRemote-control command(s):\nTRIGger:BASE:EXTA<n>:SLOPe"}, {"Level"=3, "Class Only"=FALSE, "Identifier"="RSCMXPBASE_ATTR_TRIGGER_B_SOURCE_CATALOG", "Descriptive Name"="Trigger B Source Catalog", "Data Type"=2, "Command"="TRIG:BASE:EXTB<Trigger>:CAT:SOUR?", "Access"=0, "Range Table"="", "Read Callback"="rscmxpbase_FormatTriggerRepCapString_ReadCallback.vi", "Write Callback"="rscmxpbase_FormatTriggerRepCapString_WriteCallback.vi", "Supported Models"="", "Instrument Options"="", "Flags"=0, "Help"="Lists all trigger source values that can be set using RSCMXPBASE_ATTR_TRIGGER_B_SOURCE.\n\nAvailable Repeated Capabilities:\nNone\n\nRemote-control command(s):\nTRIGger:BASE:EXTB<n>:CATalog:SOURce?"}, {"Level"=3, "Class Only"=FALSE, "Identifier"="RSCMXPBASE_ATTR_TRIGGER_B_SOURCE", "Descriptive Name"="Trigger B Source", "Data Type"=2, "Command"="TRIG:BASE:EXTB<Trigger>:SOUR", "Access"=2, "Range Table"="", "Read Callback"="rscmxpbase_FormatTriggerRepCapString_ReadCallback.vi", "Write Callback"="rscmxpbase_FormatTriggerRepCapString_WriteCallback.vi", "Supported Models"="", "Instrument Options"="", "Flags"=0, "Help"="Selects the output trigger signals to be routed to the trigger connectors. A list of all supported values can be retrieved using RSCMXPBASE_ATTR_TRIGGER_B_SOURCE_CATALOG.\n\nAvailable Repeated Capabilities:\nNone\n\nRemote-control command(s):\nTRIGger:BASE:EXTB<n>:SOURce"}, {"Level"=3, "Class Only"=FALSE, "Identifier"="RSCMXPBASE_ATTR_TRIGGER_B_DIRECTION", "Descriptive Name"="Trigger B Direction", "Data Type"=0, "Command"="TRIG:BASE:EXTB<Trigger>:DIR", "Access"=2, "Range Table"="rsCmxpBase_rngTriggerDirection", "Read Callback"="rscmxpbase_FormatTriggerRepCapInt32_ReadCallback.vi", "Write Callback"="rscmxpbase_FormatTriggerRepCapInt32_WriteCallback.vi", "Supported Models"="", "Instrument Options"="", "Flags"=0, "Help"="Configures the trigger connectors of an R&SCMW as input or output connectors.\n\nAvailable Repeated Capabilities:\nNone\n\nRemote-control command(s):\nTRIGger:BASE:EXTB<n>:DIRection"}, {"Level"=3, "Class Only"=FALSE, "Identifier"="RSCMXPBASE_ATTR_TRIGGER_B_SLOPE", "Descriptive Name"="Trigger B Slope", "Data Type"=0, "Command"="TRIG:BASE:EXTB<Trigger>:SLOP", "Access"=2, "Range Table"="rsCmxpBase_rngTriggerSlope", "Read Callback"="rscmxpbase_FormatTriggerRepCapInt32_ReadCallback.vi", "Write Callback"="rscmxpbase_FormatTriggerRepCapInt32_WriteCallback.vi", "Supported Models"="", "Instrument Options"="", "Flags"=0, "Help"="Specifies whether the rising edge or the falling edge of the trigger pulse is generated at the trigger event.\n\nThe setting applies to output trigger signals provided at the trigger connectors.\n\nAvailable Repeated Capabilities:\nNone\n\nRemote-control command(s):\nTRIGger:BASE:EXTB<n>:SLOPe"}, {"Level"=3, "Class Only"=FALSE, "Identifier"="RSCMXPBASE_ATTR_TRIGGER_C_SOURCE_CATALOG", "Descriptive Name"="Trigger C Source Catalog", "Data Type"=2, "Command"="TRIG:BASE:EXTC<Trigger>:CAT:SOUR?", "Access"=0, "Range Table"="", "Read Callback"="rscmxpbase_FormatTriggerRepCapString_ReadCallback.vi", "Write Callback"="rscmxpbase_FormatTriggerRepCapString_WriteCallback.vi", "Supported Models"="", "Instrument Options"="", "Flags"=0, "Help"="Lists all trigger source values that can be set using RSCMXPBASE_ATTR_TRIGGER_C_SOURCE.\n\nAvailable Repeated Capabilities:\nNone\n\nRemote-control command(s):\nTRIGger:BASE:EXTC<n>:CATalog:SOURce?"}, {"Level"=3, "Class Only"=FALSE, "Identifier"="RSCMXPBASE_ATTR_TRIGGER_C_SOURCE", "Descriptive Name"="Trigger C Source", "Data Type"=2, "Command"="TRIG:BASE:EXTC<Trigger>:SOUR", "Access"=2, "Range Table"="", "Read Callback"="rscmxpbase_FormatTriggerRepCapString_ReadCallback.vi", "Write Callback"="rscmxpbase_FormatTriggerRepCapString_WriteCallback.vi", "Supported Models"="", "Instrument Options"="", "Flags"=0, "Help"="Selects the output trigger signals to be routed to the trigger connectors. A list of all supported values can be retrieved using RSCMXPBASE_ATTR_TRIGGER_C_SOURCE_CATALOG.\n\nAvailable Repeated Capabilities:\nNone\n\nRemote-control command(s):\nTRIGger:BASE:EXTC<n>:SOURce"}, {"Level"=3, "Class Only"=FALSE, "Identifier"="RSCMXPBASE_ATTR_TRIGGER_C_SLOPE", "Descriptive Name"="Trigger C Slope", "Data Type"=0, "Command"="TRIG:BASE:EXTC<Trigger>:SLOP", "Access"=2, "Range Table"="rsCmxpBase_rngTriggerSlope", "Read Callback"="rscmxpbase_FormatTriggerRepCapInt32_ReadCallback.vi", "Write Callback"="rscmxpbase_FormatTriggerRepCapInt32_WriteCallback.vi", "Supported Models"="", "Instrument Options"="", "Flags"=0, "Help"="Specifies whether the rising edge or the falling edge of the trigger pulse is generated at the trigger event.\n\nThe setting applies to output trigger signals provided at the trigger connectors.\n\nAvailable Repeated Capabilities:\nNone\n\nRemote-control command(s):\nTRIGger:BASE:EXTC<n>:SLOPe"}, {"Level"=3, "Class Only"=FALSE, "Identifier"="RSCMXPBASE_ATTR_TRIGGER_D_SOURCE_CATALOG", "Descriptive Name"="Trigger D Source Catalog", "Data Type"=2, "Command"="TRIG:BASE:EXTD<Trigger>:CAT:SOUR?", "Access"=0, "Range Table"="", "Read Callback"="rscmxpbase_FormatTriggerRepCapString_ReadCallback.vi", "Write Callback"="rscmxpbase_FormatTriggerRepCapString_WriteCallback.vi", "Supported Models"="", "Instrument Options"="", "Flags"=0, "Help"="Lists all trigger source values that can be set using RSCMXPBASE_ATTR_TRIGGER_D_SOURCE.\n\nAvailable Repeated Capabilities:\nNone\n\nRemote-control command(s):\nTRIGger:BASE:EXTD<n>:CATalog:SOURce?"}, {"Level"=3, "Class Only"=FALSE, "Identifier"="RSCMXPBASE_ATTR_TRIGGER_D_SOURCE", "Descriptive Name"="Trigger D Source", "Data Type"=2, "Command"="TRIG:BASE:EXTD<Trigger>:SOUR", "Access"=2, "Range Table"="", "Read Callback"="rscmxpbase_FormatTriggerRepCapString_ReadCallback.vi", "Write Callback"="rscmxpbase_FormatTriggerRepCapString_WriteCallback.vi", "Supported Models"="", "Instrument Options"="", "Flags"=0, "Help"="Selects the output trigger signals to be routed to the trigger connectors. A list of all supported values can be retrieved using RSCMXPBASE_ATTR_TRIGGER_D_SOURCE_CATALOG.\n\nAvailable Repeated Capabilities:\nNone\n\nRemote-control command(s):\nTRIGger:BASE:EXTD<n>:SOURce"}, {"Level"=3, "Class Only"=FALSE, "Identifier"="RSCMXPBASE_ATTR_TRIGGER_D_SLOPE", "Descriptive Name"="Trigger D Slope", "Data Type"=0, "Command"="TRIG:BASE:EXTD<Trigger>:SLOP", "Access"=2, "Range Table"="rsCmxpBase_rngTriggerSlope", "Read Callback"="rscmxpbase_FormatTriggerRepCapInt32_ReadCallback.vi", "Write Callback"="rscmxpbase_FormatTriggerRepCapInt32_WriteCallback.vi", "Supported Models"="", "Instrument Options"="", "Flags"=0, "Help"="Specifies whether the rising edge or the falling edge of the trigger pulse is generated at the trigger event.\n\nThe setting applies to output trigger signals provided at the trigger connectors.\n\nAvailable Repeated Capabilities:\nNone\n\nRemote-control command(s):\nTRIGger:BASE:EXTD<n>:SLOPe"}, {"Level"=3, "Class Only"=FALSE, "Identifier"="RSCMXPBASE_ATTR_TRIGGER_E_SOURCE_CATALOG", "Descriptive Name"="Trigger E Source Catalog", "Data Type"=2, "Command"="TRIG:BASE:EXTE<Trigger>:CAT:SOUR?", "Access"=0, "Range Table"="", "Read Callback"="rscmxpbase_FormatTriggerRepCapString_ReadCallback.vi", "Write Callback"="rscmxpbase_FormatTriggerRepCapString_WriteCallback.vi", "Supported Models"="", "Instrument Options"="", "Flags"=0, "Help"="Lists all trigger source values that can be set using RSCMXPBASE_ATTR_TRIGGER_E_SOURCE\n\nAvailable Repeated Capabilities:\nNone\n\nRemote-control command(s):\nTRIGger:BASE:EXTE<n>:CATalog:SOURce?"}, {"Level"=3, "Class Only"=FALSE, "Identifier"="RSCMXPBASE_ATTR_TRIGGER_E_SOURCE", "Descriptive Name"="Trigger E Source", "Data Type"=2, "Command"="TRIG:BASE:EXTE<Trigger>:SOUR", "Access"=2, "Range Table"="", "Read Callback"="rscmxpbase_FormatTriggerRepCapString_ReadCallback.vi", "Write Callback"="rscmxpbase_FormatTriggerRepCapString_WriteCallback.vi", "Supported Models"="", "Instrument Options"="", "Flags"=0, "Help"="Selects the output trigger signals to be routed to the trigger connectors. A list of all supported values can be retrieved using RSCMXPBASE_ATTR_TRIGGER_E_SOURCE_CATALOG.\n\nAvailable Repeated Capabilities:\nNone\n\nRemote-control command(s):\nTRIGger:BASE:EXTE<n>:SOURce"}, {"Level"=3, "Class Only"=FALSE, "Identifier"="RSCMXPBASE_ATTR_TRIGGER_E_SLOPE", "Descriptive Name"="Trigger E Slope", "Data Type"=0, "Command"="TRIG:BASE:EXTE<Trigger>:SLOP", "Access"=2, "Range Table"="rsCmxpBase_rngTriggerSlope", "Read Callback"="rscmxpbase_FormatTriggerRepCapInt32_ReadCallback.vi", "Write Callback"="rscmxpbase_FormatTriggerRepCapInt32_WriteCallback.vi", "Supported Models"="", "Instrument Options"="", "Flags"=0, "Help"="Specifies whether the rising edge or the falling edge of the trigger pulse is generated at the trigger event.\n\nThe setting applies to output trigger signals provided at the trigger connectors.\n\nAvailable Repeated Capabilities:\nNone\n\nRemote-control command(s):\nTRIGger:BASE:EXTE<n>:SLOPe"}, {"Level"=2, "Class Only"=TRUE, "Identifier"="", "Descriptive Name"="Event Log", "Data Type"=0, "Command"="", "Access"=0, "Range Table"="", "Read Callback"="", "Write Callback"="", "Supported Models"="", "Instrument Options"="", "Flags"=0, "Help"="Error messages, warnings and other information are collected in the event log. It reports, for example, a state change of the network emulation or a call drop."}, {"Level"=3, "Class Only"=FALSE, "Identifier"="RSCMXPBASE_ATTR_EVENT_LOG_ALL_ENTRIES", "Descriptive Name"="Event Log All Entries", "Data Type"=6, "Command"="SENS:ELOG:ALL?", "Access"=0, "Range Table"="", "Read Callback"="", "Write Callback"="", "Supported Models"="", "Instrument Options"="", "Flags"=0, "Help"="Queries all event log entries.\n\nFor each entry, three parameters are returned: {<Severity>, <Timestamp>, <Message>}entry 1, {<Severity>, <Timestamp>, <Message>}entry 2, ...\n\nAvailable Repeated Capabilities:\nNone\n\nRemote-control command(s):\nSENSe:ELOG:ALL?"}, {"Level"=3, "Class Only"=FALSE, "Identifier"="RSCMXPBASE_ATTR_EVENT_LOG_LAST_ENTRIES", "Descriptive Name"="Event Log Last Entries", "Data Type"=6, "Command"="SENS:ELOG:LAST?", "Access"=0, "Range Table"="", "Read Callback"="", "Write Callback"="", "Supported Models"="", "Instrument Options"="", "Flags"=0, "Help"="Queries the specified number entries of the event log.\n\nAvailable Repeated Capabilities:\nNone\n\nRemote-control command(s):\nSENSe:ELOG:LAST?"}, {"Level"=3, "Class Only"=FALSE, "Identifier"="RSCMXPBASE_ATTR_HIDDEN_EVENT_LOG_SELECT_ENTRIES", "Descriptive Name"="Hidden Event Log Select Entries", "Data Type"=6, "Command"="SENS:ELOG:TIME?", "Access"=0, "Range Table"="", "Read Callback"="", "Write Callback"="", "Supported Models"="", "Instrument Options"="", "Flags"=8, "Help"="Queries all event log entries with a timestamp between <TimeStart> and <TimeEnd>.\n\nFor each relevant entry, three parameters are returned: {<Severity>, <Timestamp>, <Message>}entry 1, {<Severity>, <Timestamp>, <Message>}entry 2, ...\n\nAvailable Repeated Capabilities:\nNone\n\nRemote-control command(s):\nSENSe:ELOG:TIME?"}, {"Level"=2, "Class Only"=FALSE, "Identifier"="RSCMXPBASE_ATTR_DEVICE_ID", "Descriptive Name"="Device ID", "Data Type"=2, "Command"="SYST:DEV:ID?", "Access"=0, "Range Table"="", "Read Callback"="", "Write Callback"="", "Supported Models"="", "Instrument Options"="", "Flags"=0, "Help"="Queries the device identification of the instrument. This ID is important for ordering licenses.\n\nAvailable Repeated Capabilities:\nNone\n\nRemote-control command(s):\nSYSTem:DEVice:ID?"}, {"Level"=2, "Class Only"=FALSE, "Identifier"="RSCMXPBASE_ATTR_HIDDEN_OPTION_VERSION_INFO", "Descriptive Name"="Option Version Info", "Data Type"=2, "Command"="SYST:BASE:OPT:VERS?", "Access"=0, "Range Table"="", "Read Callback"="", "Write Callback"="", "Supported Models"="", "Instrument Options"="", "Flags"=8, "Help"="Returns version information for installed software packages. You can either query a list of all installed packages and their versions or you can query the version of a single package specified via <Application>: <Application> specified: A string is returned, indicating the version of the <Application>. If the specified <Application> is unknown / not installed, '0' is returned.<Application> omitted: A string is returned, containing a list of all installed software packages and their version in the format '<PackageName1>,<Version1>;<PackageName2>,<Version2>;...'\n\nAvailable Repeated Capabilities:\nNone\n\nRemote-control command(s):\nSYSTem:BASE:OPTion:VERSion?"}, {"Level"=2, "Class Only"=FALSE, "Identifier"="RSCMXPBASE_ATTR_HIDDEN_QUERY_OPTION_LIST", "Descriptive Name"="Query Option List", "Data Type"=6, "Command"="SYST:BASE:OPT:LIST?", "Access"=0, "Range Table"="", "Read Callback"="", "Write Callback"="", "Supported Models"="", "Instrument Options"="", "Flags"=8, "Help"="Returns a list of installed software options (licenses), hardware options, software packages and firmware applications.\nThe list can be filtered using the described parameters. If filtering results in an empty list, a '0' is returned.\nThe meaning of the filter <Validity> depends on the <OptionType> as follows:A software option is valid if there is an active license key for it. The value 'FUNCtional' is not relevant.A hardware option is functional if the corresponding hardware and all its components can be used (no defect detected). The value 'VALid' is not relevant.A firmware application is functional if the required hardware, software and license keys are available and functional. The value 'VALid' is not relevant.For software packages, the filter has no effect.\n\nAvailable Repeated Capabilities:\nNone\n\nRemote-control command(s):\nSYSTem:BASE:OPTion:LIST?"}, {"Level"=2, "Class Only"=FALSE, "Identifier"="RSCMXPBASE_ATTR_DEVICE_GROUP", "Descriptive Name"="Device Group", "Data Type"=2, "Command"="SYST:UPD:DGR", "Access"=2, "Range Table"="", "Read Callback"="", "Write Callback"="", "Supported Models"="", "Instrument Options"="", "Flags"=0, "Help"="Sets the 'Device Group' that the instrument belongs to. For remote installation, this setting must match the corresponding setting in the R&S Software Distributor options.\n\nAvailable Repeated Capabilities:\nNone\n\nRemote-control command(s):\nSYSTem:UPDate:DGRoup"}, {"Level"=2, "Class Only"=FALSE, "Identifier"="RSCMXPBASE_ATTR_COMMON_RELIABILITY", "Descriptive Name"="Common Reliability", "Data Type"=0, "Command"="SYST:BASE:REL?", "Access"=0, "Range Table"="", "Read Callback"="", "Write Callback"="", "Supported Models"="", "Instrument Options"="", "Flags"=0, "Help"="Returns a reliability value indicating errors detected by the base software.\n\nAvailable Repeated Capabilities:\nNone\n\nRemote-control command(s):\nSYSTem:BASE:RELiability?"}, {"Level"=2, "Class Only"=FALSE, "Identifier"="RSCMXPBASE_ATTR_ALL_SIGNALING_APPLICATIONS_OFF", "Descriptive Name"="All Signaling Applications Off", "Data Type"=4, "Command"="SYST:SIGN:ALL:OFF", "Access"=1, "Range Table"="", "Read Callback"="", "Write Callback"="", "Supported Models"="", "Instrument Options"="", "Flags"=0, "Help"="Switch off all signaling applications, generators or measurements.\n\nAvailable Repeated Capabilities:\nNone\n\nRemote-control command(s):\nSYSTem:SIGNaling:ALL:OFF"}, {"Level"=2, "Class Only"=FALSE, "Identifier"="RSCMXPBASE_ATTR_ALL_GENERATORS_OFF", "Descriptive Name"="All Generators Off", "Data Type"=4, "Command"="SYST:GEN:ALL:OFF", "Access"=1, "Range Table"="", "Read Callback"="", "Write Callback"="", "Supported Models"="", "Instrument Options"="", "Flags"=0, "Help"="Switch off all signaling applications, generators or measurements.\n\nAvailable Repeated Capabilities:\nNone\n\nRemote-control command(s):\nSYSTem:GENerator:ALL:OFF"}, {"Level"=2, "Class Only"=FALSE, "Identifier"="RSCMXPBASE_ATTR_ALL_MEASUREMENTS_OFF", "Descriptive Name"="All Measurements Off", "Data Type"=4, "Command"="SYST:MEAS:ALL:OFF", "Access"=1, "Range Table"="", "Read Callback"="", "Write Callback"="", "Supported Models"="", "Instrument Options"="", "Flags"=0, "Help"="Switch off all signaling applications, generators or measurements.\n\nAvailable Repeated Capabilities:\nNone\n\nRemote-control command(s):\nSYSTem:MEASurement:ALL:OFF"}, {"Level"=1, "Class Only"=TRUE, "Identifier"="", "Descriptive Name"="File", "Data Type"=0, "Command"="", "Access"=0, "Range Table"="", "Read Callback"="", "Write Callback"="", "Supported Models"="", "Instrument Options"="", "Flags"=0, "Help"="Contains functionality for managing files."}, {"Level"=2, "Class Only"=FALSE, "Identifier"="RSCMXPBASE_ATTR_FILE_MANAGER_ALIASES", "Descriptive Name"="File Manager Aliases", "Data Type"=2, "Command"="MMEM:ALI?", "Access"=0, "Range Table"="", "Read Callback"="", "Write Callback"="", "Supported Models"="", "Instrument Options"="", "Flags"=0, "Help"="Returns the defined alias entries and the assigned directories. These settings are predefined and cannot be configured.\n\nAvailable Repeated Capabilities:\nNone\n\nRemote-control command(s):\nMMEMory:ALIases?"}, {"Level"=2, "Class Only"=FALSE, "Identifier"="RSCMXPBASE_ATTR_SET_FILE_ATTRIBUTE", "Descriptive Name"="Set File Attribute", "Data Type"=6, "Command"="MMEM:ATTR", "Access"=1, "Range Table"="", "Read Callback"="", "Write Callback"="", "Supported Models"="", "Instrument Options"="", "Flags"=0, "Help"="Sets file attributes for files and directories.\n\nAvailable Repeated Capabilities:\nNone\n\nRemote-control command(s):\nMMEMory:ATTRibute"}, {"Level"=2, "Class Only"=FALSE, "Identifier"="RSCMXPBASE_ATTR_HIDDEN_QUERY_FILE_ATTRIBUTE", "Descriptive Name"="Query File Attribute", "Data Type"=6, "Command"="MMEM:ATTR?", "Access"=0, "Range Table"="", "Read Callback"="", "Write Callback"="", "Supported Models"="", "Instrument Options"="", "Flags"=8, "Help"="Queries file attributes for files and directories.\n\nAvailable Repeated Capabilities:\nNone\n\nRemote-control command(s):\nMMEMory:ATTRibute?"}, {"Level"=2, "Class Only"=FALSE, "Identifier"="RSCMXPBASE_ATTR_HIDDEN_QUERY_DIRECTORY_CONTENTS", "Descriptive Name"="Query Directory Contents", "Data Type"=6, "Command"="MMEM:CAT?", "Access"=0, "Range Table"="", "Read Callback"="", "Write Callback"="", "Supported Models"="", "Instrument Options"="", "Flags"=8, "Help"="Returns information on the contents of the current or of a specified directory.\n\nAvailable Repeated Capabilities:\nNone\n\nRemote-control command(s):\nMMEMory:CATalog?"}, {"Level"=2, "Class Only"=FALSE, "Identifier"="RSCMXPBASE_ATTR_HIDDEN_QUERY_SUBDIRECTORIES", "Descriptive Name"="Query Subdirectories", "Data Type"=6, "Command"="MMEM:DCAT?", "Access"=0, "Range Table"="", "Read Callback"="", "Write Callback"="", "Supported Models"="", "Instrument Options"="", "Flags"=8, "Help"="Returns the subdirectories of the current or of a specified directory.\n\nAvailable Repeated Capabilities:\nNone\n\nRemote-control command(s):\nMMEMory:DCATalog?"}, {"Level"=2, "Class Only"=FALSE, "Identifier"="RSCMXPBASE_ATTR_HIDDEN_QUERY_SUBDIRECTORY_COUNT", "Descriptive Name"="Query Subdirectory Count", "Data Type"=0, "Command"="MMEM:DCAT:LENG?", "Access"=0, "Range Table"="", "Read Callback"="", "Write Callback"="", "Supported Models"="", "Instrument Options"="", "Flags"=8, "Help"="Returns the number of subdirectories of the current or of a specified directory. The number includes the directory strings '.' and '..' so that it corresponds to the number of strings returned by the MMEMory:DCATalog? command.\n\nAvailable Repeated Capabilities:\nNone\n\nRemote-control command(s):\nMMEMory:DCATalog:LENGth?"}, {"Level"=2, "Class Only"=FALSE, "Identifier"="RSCMXPBASE_ATTR_HIDDEN_QUERY_DIRECTORY_PATH_COUNT", "Descriptive Name"="Query Directory Path Count", "Data Type"=0, "Command"="MMEM:CAT:LENG?", "Access"=0, "Range Table"="", "Read Callback"="", "Write Callback"="", "Supported Models"="", "Instrument Options"="", "Flags"=8, "Help"="Returns the number of files and subdirectories of the current or of a specified directory. The number includes the directory strings '.' and '..' so that it corresponds to the number of strings returned by the MMEMory:CATalog? command after the initial numeric parameters.\n\nAvailable Repeated Capabilities:\nNone\n\nRemote-control command(s):\nMMEMory:CATalog:LENGth?"}, {"Level"=2, "Class Only"=FALSE, "Identifier"="RSCMXPBASE_ATTR_EDIT_PATH", "Descriptive Name"="Edit Path", "Data Type"=2, "Command"="MMEM:CDIR", "Access"=2, "Range Table"="", "Read Callback"="", "Write Callback"="", "Supported Models"="", "Instrument Options"="", "Flags"=0, "Help"="Changes the current directory for mass memory storage. If <DirectoryName> is omitted, the current directory is set to '\\'.\n\nAvailable Repeated Capabilities:\nNone\n\nRemote-control command(s):\nMMEMory:CDIRectory"}, {"Level"=2, "Class Only"=FALSE, "Identifier"="RSCMXPBASE_ATTR_MOVE", "Descriptive Name"="Move", "Data Type"=6, "Command"="MMEM:MOVE", "Access"=1, "Range Table"="", "Read Callback"="", "Write Callback"="", "Supported Models"="", "Instrument Options"="", "Flags"=0, "Help"="Moves or renames an existing object (file or directory) to a new location.\n\nAvailable Repeated Capabilities:\nNone\n\nRemote-control command(s):\nMMEMory:MOVE"}, {"Level"=2, "Class Only"=FALSE, "Identifier"="RSCMXPBASE_ATTR_COPY_FILE", "Descriptive Name"="Copy File", "Data Type"=6, "Command"="MMEM:COPY", "Access"=1, "Range Table"="", "Read Callback"="", "Write Callback"="", "Supported Models"="", "Instrument Options"="", "Flags"=0, "Help"="Copies an existing file. The target directory must exist.\n\nAvailable Repeated Capabilities:\nNone\n\nRemote-control command(s):\nMMEMory:COPY"}, {"Level"=2, "Class Only"=FALSE, "Identifier"="RSCMXPBASE_ATTR_DELETE_FILE", "Descriptive Name"="Delete File", "Data Type"=2, "Command"="MMEM:DEL", "Access"=1, "Range Table"="", "Read Callback"="", "Write Callback"="", "Supported Models"="", "Instrument Options"="", "Flags"=0, "Help"="Deletes the specified files.\n\nAvailable Repeated Capabilities:\nNone\n\nRemote-control command(s):\nMMEMory:DELete"}, {"Level"=2, "Class Only"=FALSE, "Identifier"="RSCMXPBASE_ATTR_DELETE_DIRECTORY", "Descriptive Name"="Delete Directory", "Data Type"=2, "Command"="MMEM:RDIR", "Access"=1, "Range Table"="", "Read Callback"="", "Write Callback"="", "Supported Models"="", "Instrument Options"="", "Flags"=0, "Help"="Removes an existing empty directory from the mass memory storage system.\n\nAvailable Repeated Capabilities:\nNone\n\nRemote-control command(s):\nMMEMory:RDIRectory"}, {"Level"=2, "Class Only"=FALSE, "Identifier"="RSCMXPBASE_ATTR_CREATE_DIRECTORY", "Descriptive Name"="Create Directory", "Data Type"=2, "Command"="MMEM:MDIR", "Access"=1, "Range Table"="", "Read Callback"="", "Write Callback"="", "Supported Models"="", "Instrument Options"="", "Flags"=0, "Help"="Creates a directory. If necessary, an entire path consisting of several subdirectories is created.\n\nAvailable Repeated Capabilities:\nNone\n\nRemote-control command(s):\nMMEMory:MDIRectory"}, {"Level"=2, "Class Only"=FALSE, "Identifier"="RSCMXPBASE_ATTR_CHANGE_DRIVE", "Descriptive Name"="Change Drive", "Data Type"=2, "Command"="MMEM:MSIS", "Access"=2, "Range Table"="", "Read Callback"="", "Write Callback"="", "Supported Models"="", "Instrument Options"="", "Flags"=0, "Help"="Changes the default storage unit (drive or server) for mass memory storage. When the default storage unit is changed, it is checked whether the current directory (see RSCMXPBASE_ATTR_EDIT_PATH) is also available on the new storage unit. If not, the current directory is automatically set to '\\'.\n\nAvailable Repeated Capabilities:\nNone\n\nRemote-control command(s):\nMMEMory:MSIS"}, {"Level"=2, "Class Only"=FALSE, "Identifier"="RSCMXPBASE_ATTR_WRITE_FROM_FILE_TO_INSTRUMENT", "Descriptive Name"="Write From File To Instrument", "Data Type"=6, "Command"="MMEM:DATA", "Access"=1, "Range Table"="", "Read Callback"="", "Write Callback"="", "Supported Models"="", "Instrument Options"="", "Flags"=0, "Help"="Stores the specified block data into the specified file.\n\nAvailable Repeated Capabilities:\nNone\n\nRemote-control command(s):\nMMEMory:DATA"}, {"Level"=2, "Class Only"=FALSE, "Identifier"="RSCMXPBASE_ATTR_HIDDEN_READ_TO_FILE_FROM_INSTRUMENT", "Descriptive Name"="Read To File From Instrument", "Data Type"=2, "Command"="MMEM:DATA?", "Access"=0, "Range Table"="", "Read Callback"="", "Write Callback"="", "Supported Models"="", "Instrument Options"="", "Flags"=8, "Help"="Queries the specified block data into the specified file.\n\nAvailable Repeated Capabilities:\nNone\n\nRemote-control command(s):\nMMEMory:DATA?"}, {"Level"=2, "Class Only"=FALSE, "Identifier"="RSCMXPBASE_ATTR_QUERY_DRIVES_LIST", "Descriptive Name"="Query Drives List", "Data Type"=2, "Command"="MMEM:DRIV?", "Access"=0, "Range Table"="", "Read Callback"="", "Write Callback"="", "Supported Models"="", "Instrument Options"="", "Flags"=0, "Help"="Returns a list of the available drives.\n\nAvailable Repeated Capabilities:\nNone\n\nRemote-control command(s):\nMMEMory:DRIVes?"}, {"Level"=2, "Class Only"=FALSE, "Identifier"="RSCMXPBASE_ATTR_DATA_SET_APPLICATION_RESTORE", "Descriptive Name"="Data Set Application Restore", "Data Type"=6, "Command"="MMEM:LOAD:ITEM", "Access"=1, "Range Table"="", "Read Callback"="", "Write Callback"="", "Supported Models"="", "Instrument Options"="", "Flags"=0, "Help"="Executes a partial recall. That means, restores a selected part of a save file. You can restore all settings of a specific application instance. Or you can restore the list mode settings of a specific measurement application instance.\n\nAvailable Repeated Capabilities:\nNone\n\nRemote-control command(s):\nMMEMory:LOAD:ITEM"}, {"Level"=2, "Class Only"=FALSE, "Identifier"="RSCMXPBASE_ATTR_DATA_SET_APPLICATION_SAVE", "Descriptive Name"="Data Set Application Save", "Data Type"=6, "Command"="MMEM:STOR:ITEM", "Access"=1, "Range Table"="", "Read Callback"="", "Write Callback"="", "Supported Models"="", "Instrument Options"="", "Flags"=0, "Help"="Executes a partial save, i.e. stores a part of the instrument settings to the specified file. You can store all settings of a specific application instance. Or you can store the list mode settings of a specific measurement application instance.\n\nAvailable Repeated Capabilities:\nNone\n\nRemote-control command(s):\nMMEMory:STORe:ITEM"}, {"Level"=2, "Class Only"=FALSE, "Identifier"="RSCMXPBASE_ATTR_STORE_INSTRUMENT_SETTINGS", "Descriptive Name"="Store Instrument Settings", "Data Type"=2, "Command"="MMEM:SAV", "Access"=1, "Range Table"="", "Read Callback"="", "Write Callback"="", "Supported Models"="", "Instrument Options"="", "Flags"=0, "Help"="Stores the current instrument settings to the specified file.\n\nAvailable Repeated Capabilities:\nNone\n\nRemote-control command(s):\nMMEMory:SAV"}, {"Level"=2, "Class Only"=FALSE, "Identifier"="RSCMXPBASE_ATTR_LOAD_INSTRUMENT_SETTINGS", "Descriptive Name"="Load Instrument Settings", "Data Type"=2, "Command"="MMEM:RCL", "Access"=1, "Range Table"="", "Read Callback"="", "Write Callback"="", "Supported Models"="", "Instrument Options"="", "Flags"=0, "Help"="Recalls the current instrument settings to the specified file.\n\nAvailable Repeated Capabilities:\nNone\n\nRemote-control command(s):\nMMEMory:RCL"}, {"Level"=1, "Class Only"=TRUE, "Identifier"="", "Descriptive Name"="Utility", "Data Type"=0, "Command"="", "Access"=0, "Range Table"="", "Read Callback"="", "Write Callback"="", "Supported Models"="", "Instrument Options"="", "Flags"=0, "Help"="General Utilitity attributes.\n\n(1) System Version:\nGets system version.\n\n(2) System Error:\nThis attribute queries the earliest entry in the error queue, and deletes it after the readout.\n\n(3) System All Errors:\nReads all errors from instrument.\n\n(4) System Preset:\nResets instrument."}, {"Level"=2, "Class Only"=FALSE, "Identifier"="RSCMXPBASE_ATTR_HIDDEN_AMBIENT_TEMPERATURE", "Descriptive Name"="Hidden Ambient Temperature", "Data Type"=6, "Command"="SENS:BASE:TEMP:OPER:AMB?", "Access"=0, "Range Table"="", "Read Callback"="", "Write Callback"="", "Supported Models"="", "Instrument Options"="", "Flags"=8, "Help"="Queries the ambient temperature measured via a sensor in the instrument.\n\nAmbient temperatures reported by self-tests are also measured via this sensor.\n\nAvailable Repeated Capabilities:\nNone\n\nRemote-control command(s):\nSENSe:BASE:TEMPerature:OPERating:AMBient?"}, {"Level"=2, "Class Only"=FALSE, "Identifier"="RSCMXPBASE_ATTR_HIDDEN_SYSTEM_DATA_FORMAT", "Descriptive Name"="Hidden System Data Format", "Data Type"=6, "Command"="FORM:BASE", "Access"=2, "Range Table"="", "Read Callback"="", "Write Callback"="", "Supported Models"="", "Instrument Options"="", "Flags"=8, "Help"="Selects the format for numeric data transferred to and from the R&SCMX500, for example query results.\n\nAvailable Repeated Capabilities:\nNone\n\nRemote-control command(s):\nFORMat:BASE[:DATA]"}, {"Level"=2, "Class Only"=FALSE, "Identifier"="RSCMXPBASE_ATTR_HIDDEN_SYSTEM_DATE", "Descriptive Name"="Hidden System Date", "Data Type"=6, "Command"="SYST:DATE", "Access"=2, "Range Table"="", "Read Callback"="", "Write Callback"="", "Supported Models"="", "Instrument Options"="", "Flags"=8, "Help"="Sets the UTC date of the operating system calendar.\n\nAvailable Repeated Capabilities:\nNone\n\nRemote-control command(s):\nSYSTem:DATE[:UTC]"}, {"Level"=2, "Class Only"=FALSE, "Identifier"="RSCMXPBASE_ATTR_HIDDEN_SYSTEM_TIME", "Descriptive Name"="Hidden System Time", "Data Type"=6, "Command"="SYST:TIME", "Access"=2, "Range Table"="", "Read Callback"="", "Write Callback"="", "Supported Models"="", "Instrument Options"="", "Flags"=8, "Help"="Sets the universal time coordinated (UTC) of the operating system clock.\n\nAvailable Repeated Capabilities:\nNone\n\nRemote-control command(s):\nSYSTem:TIME[:UTC]"}, {"Level"=2, "Class Only"=FALSE, "Identifier"="RSCMXPBASE_ATTR_HIDDEN_SYSTEM_INSTRUMENT_FOOTPRINT", "Descriptive Name"="Hidden System Instrument Footprint", "Data Type"=2, "Command"="SYST:DFPR?", "Access"=0, "Range Table"="", "Read Callback"="", "Write Callback"="", "Supported Models"="", "Instrument Options"="", "Flags"=8, "Help"="Generates an XML file with footprint information about the instrument.\n\nAvailable Repeated Capabilities:\nNone\n\nRemote-control command(s):\nSYSTem:DFPRint?"}, {"Level"=2, "Class Only"=FALSE, "Identifier"="RSCMXPBASE_ATTR_SYSTEM_VERSION", "Descriptive Name"="System Version", "Data Type"=2, "Command"="SYST:VERSion?", "Access"=0, "Range Table"="", "Read Callback"="", "Write Callback"="", "Supported Models"="", "Instrument Options"="", "Flags"=0, "Help"="Gets system version.\n\nAvailable Repeated Capabilities:\nNone\n\nRemote-control command(s):\nSYSTem:VERSion?"}, {"Level"=2, "Class Only"=FALSE, "Identifier"="RSCMXPBASE_ATTR_SYSTEM_ERROR", "Descriptive Name"="System Error", "Data Type"=2, "Command"="SYST:ERRor?", "Access"=0, "Range Table"="", "Read Callback"="", "Write Callback"="", "Supported Models"="", "Instrument Options"="", "Flags"=0, "Help"="This attribute queries the earliest entry in the error queue, and deletes it after the readout.\n\nAvailable Repeated Capabilities:\nNone\n\nRemote-control command(s):\nSYSTem:ERRor?"}, {"Level"=2, "Class Only"=FALSE, "Identifier"="RSCMXPBASE_ATTR_SYSTEM_ALL_ERRORS", "Descriptive Name"="System All Errors", "Data Type"=2, "Command"="SYST:ERR:ALL?", "Access"=0, "Range Table"="", "Read Callback"="", "Write Callback"="", "Supported Models"="", "Instrument Options"="", "Flags"=0, "Help"="Reads all errors from instrument.\n\nAvailable Repeated Capabilities:\nNone\n\nRemote-control command(s):\nSYSTem:ERRor:ALL?"}, {"Level"=2, "Class Only"=FALSE, "Identifier"="RSCMXPBASE_ATTR_SYSTEM_RESET", "Descriptive Name"="System Reset", "Data Type"=4, "Command"="*RST", "Access"=1, "Range Table"="", "Read Callback"="", "Write Callback"="", "Supported Models"="", "Instrument Options"="", "Flags"=0, "Help"="Resets all applications.\n\nAvailable Repeated Capabilities:\nNone\n\nRemote-control command(s):\n*RST"}, {"Level"=2, "Class Only"=FALSE, "Identifier"="RSCMXPBASE_ATTR_SYSTEM_RESET_ALL", "Descriptive Name"="System Reset All", "Data Type"=4, "Command"="SYST:RES:ALL", "Access"=1, "Range Table"="", "Read Callback"="", "Write Callback"="", "Supported Models"="", "Instrument Options"="", "Flags"=0, "Help"="Resets the entire instrument, including base settings and all applications, even applications of other than the used remote channel.\n\nAvailable Repeated Capabilities:\nNone\n\nRemote-control command(s):\nSYSTem:RESet:ALL"}, {"Level"=2, "Class Only"=FALSE, "Identifier"="RSCMXPBASE_ATTR_SYSTEM_RESET_BASE_SETTINGS", "Descriptive Name"="System Reset Base Settings", "Data Type"=4, "Command"="SYST:RES:BASE", "Access"=1, "Range Table"="", "Read Callback"="", "Write Callback"="", "Supported Models"="", "Instrument Options"="", "Flags"=0, "Help"="Resets the base settings.\n\nAvailable Repeated Capabilities:\nNone\n\nRemote-control command(s):\nSYSTem:RESet:BASE"}, {"Level"=2, "Class Only"=FALSE, "Identifier"="RSCMXPBASE_ATTR_SYSTEM_ALL_ERROR_CODES", "Descriptive Name"="System All Error Codes", "Data Type"=6, "Command"="SYST:ERR:CODE:ALL?", "Access"=0, "Range Table"="", "Read Callback"="", "Write Callback"="", "Supported Models"="", "Instrument Options"="", "Flags"=0, "Help"="Queries and deletes all entries in the error queue.\n\nAvailable Repeated Capabilities:\nNone\n\nRemote-control command(s):\nSYSTem:ERRor:CODE:ALL?"}, {"Level"=2, "Class Only"=FALSE, "Identifier"="RSCMXPBASE_ATTR_SYSTEM_ERROR_CODE", "Descriptive Name"="System Error Code", "Data Type"=0, "Command"="SYST:ERR:CODE?", "Access"=0, "Range Table"="", "Read Callback"="", "Write Callback"="", "Supported Models"="", "Instrument Options"="", "Flags"=0, "Help"="Queries and deletes the oldest entry in the error queue.\n\nAvailable Repeated Capabilities:\nNone\n\nRemote-control command(s):\nSYSTem:ERRor:CODE[:NEXT]?"}, {"Level"=2, "Class Only"=FALSE, "Identifier"="RSCMXPBASE_ATTR_SYSTEM_ERROR_QUEUE_COUNT", "Descriptive Name"="System Error Queue Count", "Data Type"=0, "Command"="SYST:ERR:COUN?", "Access"=0, "Range Table"="", "Read Callback"="", "Write Callback"="", "Supported Models"="", "Instrument Options"="", "Flags"=0, "Help"="Queries the number of entries in the error queue.\n\nAvailable Repeated Capabilities:\nNone\n\nRemote-control command(s):\nSYSTem:ERRor:COUNt?"}, {"Level"=2, "Class Only"=FALSE, "Identifier"="RSCMXPBASE_ATTR_CONFIGURE_UPDATE_ON_REMOTE", "Descriptive Name"="Configure Update On Remote", "Data Type"=3, "Command"="SYST:DISP:UPD", "Access"=2, "Range Table"="", "Read Callback"="", "Write Callback"="", "Supported Models"="", "Instrument Options"="", "Flags"=0, "Help"="Defines whether the display shall be updated or not while the instrument is in the remote state. If the display (update) is switched off, the normal GUI is replaced by a static image while the instrument is in the remote state. Switching off the display can speed up the measurement. This is the recommended state.\n\nAvailable Repeated Capabilities:\nNone\n\nRemote-control command(s):\nSYSTem:DISPlay:UPDate"}] {"Flags" format="%08b"; "Access" items=["Read Only", "Write Only", "Read/Write"]; "Data Type" items=["Integer 32", "Double", "String", "Boolean", "None", "Integer 64", "RawString"]}
  in  "Supported Models":string[](array[string])=["CMX", "CMP", "CMW", "PVT"]
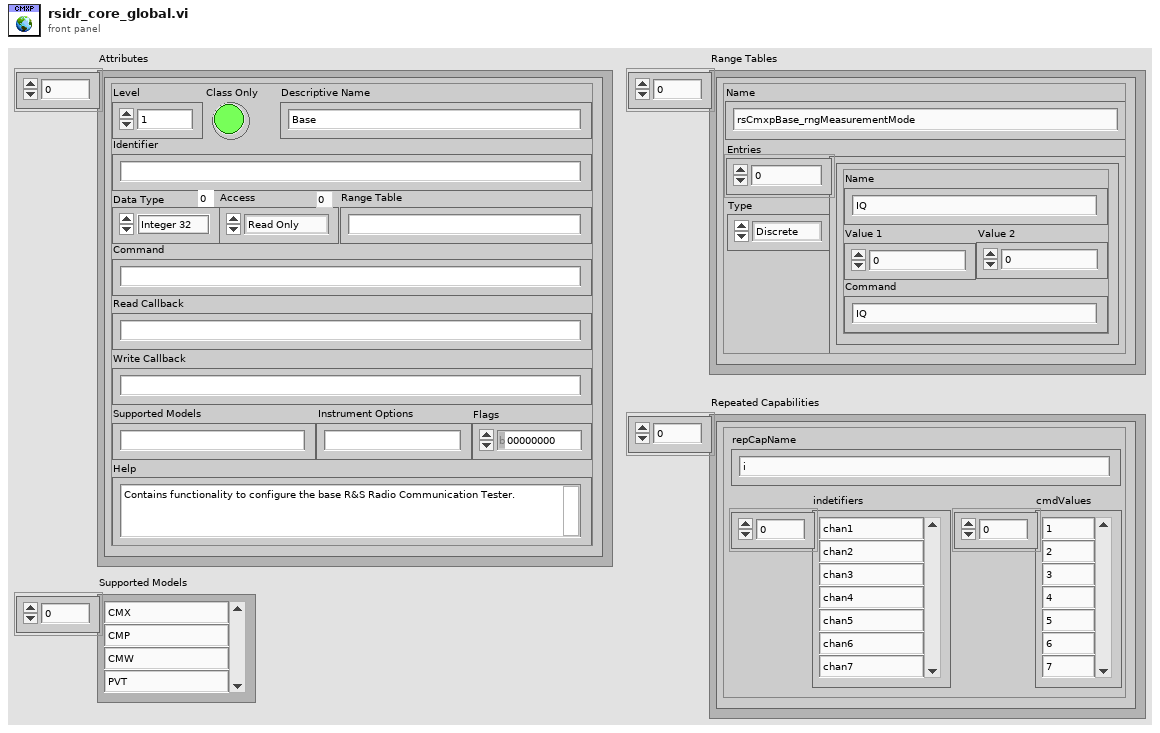
[diagram p1: front panel]
types:
  T1 = typedef "Rohde&Schwarz CMXP Base.lvlib/rsidr_core.lvlib/type_Input_Format_RepCap.ctl" = cluster{"repCapName":string, "indetifiers":string[], "cmdValues":string[]}
  T2 = typedef "Rohde&Schwarz CMXP Base.lvlib/rsidr_core.lvlib/type_Input_Format_RangeTable.ctl" = cluster{"Type":u16, "Name":string, "Entries":cluster{"Name":string, "Value 1":dbl, "Value 2":dbl, "Command":string}[]}
  T3 = typedef "Rohde&Schwarz CMXP Base.lvlib/rsidr_core.lvlib/type_Input_Format_Attribute.ctl" = cluster{"Level":i32, "Class Only":bool, "Identifier":string, "Descriptive Name":string, "Data Type":u16, "Command":string, "Access":u16, "Range Table":string, "Read Callback":string, "Write Callback":string, "Supported Models":string, "Instrument Options":string, "Flags":i32, "Help":string}
diagram:
